vi "Filter Wheel GUI.vi"(9 "Standalone":bool=TRUE, 10 "Init Data":variant, 11 "Filter Wheel name":string="Default") -> ()   [LabVIEW 2021]
uses:
  Filter Wheel Arduino Control/Filter Wheel Arduino Command cluster.ctl
  typedefs/CC enum Operation Mode.ctl
  Filter Wheel Arduino Control/Filter Wheel Arduino Homing cluster.ctl
  Filter Wheel Object/Filter Wheel.lvclass
  Filter Wheel configuration.ctl
  Filter Wheel Object/Filter Wheel Details.ctl
  Subsystems/SS typedef cluster Instrument Command Queue Data.ctl
  Subsystems/SS cluster Data Queue type.ctl
  FW cmd Q Move Parameters.ctl
  <vilib>/Utility/miscctls.llb/LVRowAndColumnTypeDef.ctl
  FW cluster Status.ctl
  FW enum status.ctl
  Filter Wheel Object/Filter Wheel.lvclass/Filter Wheel.ctl
  hk-channel-class/HK Item/HK Channel Units and Setup.ctl
  hk-channel-class/HK Item/HK Channel enum Data Type.ctl
  hk-channel-class/HK Item/HK Item.lvclass
  hk-channel-class/HK Item/HK Channel cluster Telemetry Data.ctl
  FW cmd Q Move Position Parameters.ctl
  typedefs/CC cluster Alarm Data.ctl
  Filter Wheel Simulator/Filter Wheel Simulator.lvclass
  C:/Development/prime/Prime-RIMAS/Filter Wheel/Filter Wheel Object/Filter Wheel.lvclass
  Filter Wheel Simulator/Filter Wheel Simulator.lvclass/Filter Wheel Simulator.ctl
  Filter Wheel Arduino Control/FW Arduino Control.lvclass
panel:
  out "Messages":string
  in  "Mode":T1
  in  "Tab Control":T2(tab)
  out "Wheel Name":string
  out "Moving Message":string="Filter Wheel Moving...."
  in  "Error":bool
  out "Homed":bool[](array[boolean])
  in  "Wheel To Home":u16(ring) items=["InnerWheel", "OuterWheel"]
  in  "STOP":bool
  out "Connected":bool
  in  "Filter Wheel Displays":T3 {"Gauge 0" scale=0.0..3.0; "Gauge 4" scale=0.0..7.0; "Gauge 3" scale=0.0..5.0; "Gauge 2" scale=0.0..3.0; "Gauge 5" scale=0.0..32768.0; "Gauge 8" scale=0.0..32768.0; "Gauge 6" scale=0.0..32768.0; "Gauge 7" scale=0.0..32768.0}
  in  "Home":bool
  in  "Alarms?":bool=TRUE
  in  "Default Speed":u16=200 min=20 max=4000 step=10
  in  "Movement Parameters":T4
  in  "Sim Velocity (steps/sec)":i32
  in  "Connect":bool
  in  "Serial Port":refnum<visa-resource-name>="COM11"
  in  "Simulate":bool
  in  "Close":bool
  in  "Filter Wheel Table":cluster{i32[], "Dir":bool}[][](array[cluster])=[[{[], "Dir"=TRUE}, {[2800], "Dir"=TRUE}, {[2800, 2800], "Dir"=TRUE}, {[950, 1850], "Dir"=FALSE}], [{[2800], "Dir"=FALSE}, {[], "Dir"=TRUE}, {[2800], "Dir"=TRUE}, {[2800, 2800], "Dir"=TRUE}], [{[2800, 2800], "Dir"=FALSE}, {[2800], "Dir"=FALSE}, {[], "Dir"=TRUE}, {[2800], "Dir"=TRUE}], [{[2800, 2800], "Dir"=TRUE}, {[2800, 2800], "Dir"=FALSE}, {[2800], "Dir"=FALSE}, {[], "Dir"=TRUE}]]
  in  "Open Arduino Log":bool
  out "Moving":bool[](array[boolean])
  out "Last Move Positions":u32[](array[numeric])
  out "On the notch":bool[](array[boolean])
  in  "Filter Wheel Settings":T5={"Direction"=TRUE, "NUMBER OF  STEPS"=2900, "SPEED STEPS/SEC"=200, "ACC/DECEL STEPS/SEC^2"=4000, "Move mode"=0, "EN/DIS?"=TRUE, "delay before \nread (ms)"=750, "Timeout before \nstop (ms)"=13000} {"Move mode" items=["Relative steps ##", "Search switch"]; "ACC/DECEL STEPS/SEC^2" max=4000; "SPEED STEPS/SEC" min=20 max=4000 step=10}
  in  "MOTOR NUMBER":u8 max=3 step=1
  in  "Command Preview":string
  out "Response":string
  in  "Send Command":bool
  in  "Read":bool
  in  "Restore Defaults":bool
  in  "Remove Pos":bool
  in  "Add Pos":bool
  in  "Save Button":bool
  in  "Remove Fw":bool
  in  "Add Fw":bool
  in  "Wheels":i32(listbox)
  in  "Positions":i32(listbox)
  # "Click for info"
  # "Invalid combos defined here"
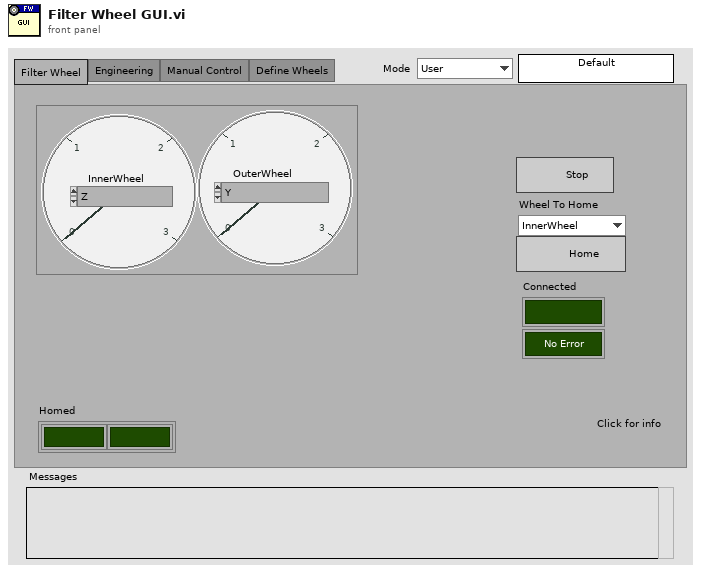
[diagram p1: front panel]
types:
  T1 = typedef "CC enum Operation Mode.ctl" = enum16{"User", "Engineering"}
  T2 = enum32{"Filter Wheel", "Engineering", "Manual Control", "Define Wheels"}
  T3 = cluster{"Gauge 0":i32, "Gauge 2":i32, "Gauge 3":i32, "Gauge 4":i32, "Gauge 5":i32, "Gauge 6":i32, "Gauge 7":i32, "Gauge 8":i32, "Position 0":i32, "Position 1":i32, "Position 2":i32, "Position 3":i32}
  T4 = typedef "Filter Wheel Arduino Homing cluster.ctl" = cluster{"Direction (F: CW)":bool, "Speed":i32, "Accel":i32, "Min Distance":i32, "Short Leg":i32, "Error Cnts":i32}
  T5 = typedef "Filter Wheel Arduino Command cluster.ctl" = cluster{"Direction":bool, "NUMBER OF  STEPS":u32, "SPEED STEPS/SEC":u16, "ACC/DECEL STEPS/SEC^2":u16, "Move mode":u16, "EN/DIS?":bool, "delay before \nread (ms)":u32, "Timeout before \nstop (ms)":u32}
  T6 = typedef "SS typedef cluster Instrument Command Queue Data.ctl" = cluster{"Cmd":string, "Parameters":variant}
  T7 = typedef "Filter Wheel.lvclass/Filter Wheel configuration.ctl" = cluster{"Num Wheels":i32, "Filters":T8[], "Invalid Combinations":i32[][], "Addr":refnum<visa-resource-name>, "Name":string, "Simulate":bool, "Homing Parameters":T4, "Default Speed":u16}
  T8 = typedef "Filter Wheel.lvclass/Filter Wheel Details.ctl" = cluster{"Names":string[], "Relative Position":i32[], "Wheel Name":string}
  T9 = typedef "FW cmd Q Move Parameters.ctl" = cluster{"Wheel ID":i32, "Position":i32}
  T10 = typedef "LVRowAndColumnTypeDef.ctl" = cluster{"Row":i32, "Column":i32}
  T11 = typedef "FW cluster Status.ctl" = cluster{"State":T12, "Positions":i32[], "Names":string[], "Notch":bool[], "Moving":bool[]}
  T12 = typedef "FW enum status.ctl" = enum16{"Initializing", "Moving", "Move Complete", "Error"}
  T13 = cluster{"state":refnum<user-event>, "Filter Wheel ref":refnum<class "Filter Wheel.lvclass">, "Filter Wheel Info":T7, "FW names":string[], "Pos Names":cluster{"Table":string[][]}[], "cmd q":refnum<queue>, "Cmd":T6, "Data Q":refnum<queue>, "Move":T9, "error":errorcluster, "next poll":timestamp, "FW refs":refnum<vi>[], "Wheel":i32, "Coords":T10, "Motor #":u8, "fw name":string, "Simulate":bool, "ch names":string[][], "FW Status":T11, "Error State":string, "Name":string, "Period":dbl}
  T14 = typedef "HK Item.lvclass/HK Channel Units and Setup.ctl" = cluster{"Unit Type":string, "Units":string, "Configuration":string, "Digits":i32, "Data Type":T15, "Exponential?":bool, "Source":string}
  T15 = typedef "HK Item.lvclass/HK Channel enum Data Type.ctl" = enum16{"Floating Point", "Integer", "Enum", "String", "Waveform", "File"}
  T16 = typedef "SS cluster Data Queue type.ctl" = cluster{"Source":string, "Type":string, "Data":variant}
  T17 = typedef "FW cmd Q Move Position Parameters.ctl" = cluster{"Position Names":string[]}
  T18 = enum32{"Page Enabled", "Page Disabled", "Page Disabled & Grayed"}
  T19 = typedef "CC cluster Alarm Data.ctl" = cluster{"Measured Value":dbl, "Alarm Low":dbl, "Alarm High":dbl, "Message":string, "Source":string}
  T20 = typedef "HK Item.lvclass/HK Channel cluster Telemetry Data.ctl" = cluster{"Ch Names":string[], "Ch Values":dbl[], "Timestamp":timestamp, "Data Type":T15}
  T21 = cluster{"Gauge 0":bool, "Gauge 2":bool, "Gauge 3":bool, "Gauge 4":bool, "Gauge 5":bool, "Gauge 6":bool, "Gauge 7":bool, "Gauge 8":bool, "Position 0":bool, "Position 1":bool, "Position 2":bool, "Position 3":bool}
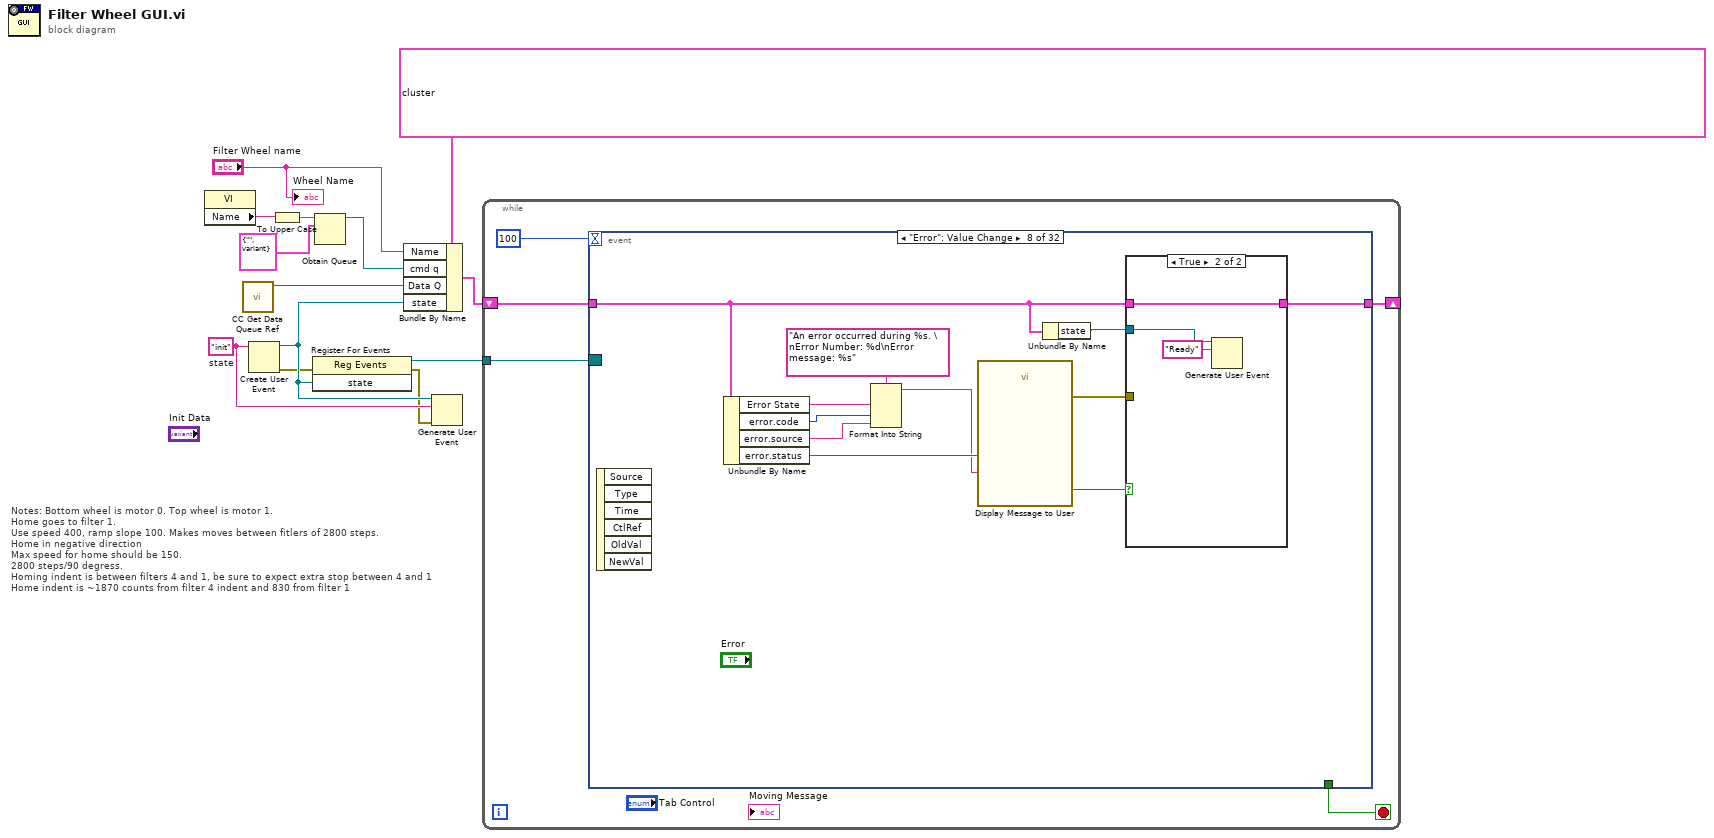
[diagram p0: block diagram]
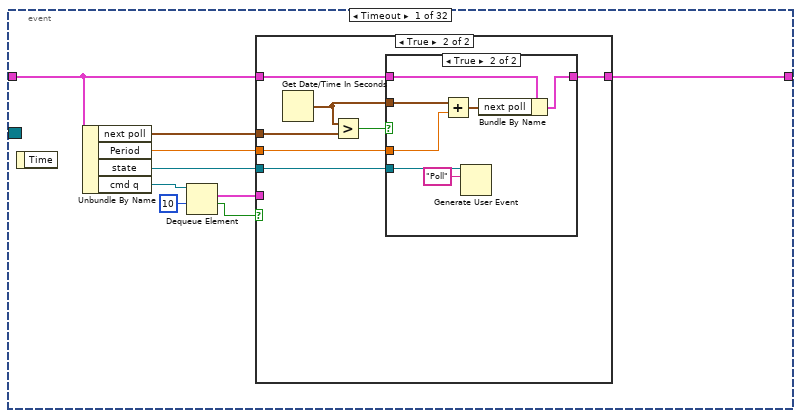
[diagram p2: hidden frame]
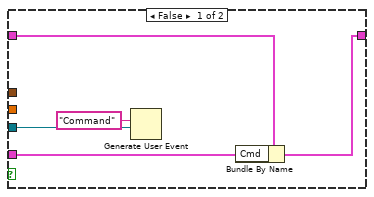
[diagram p3: hidden frame]
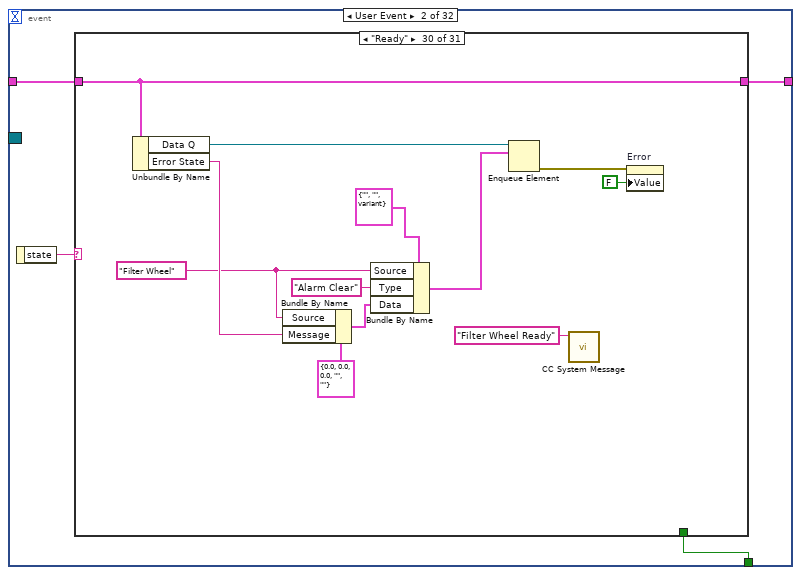
[diagram p5: hidden frame]
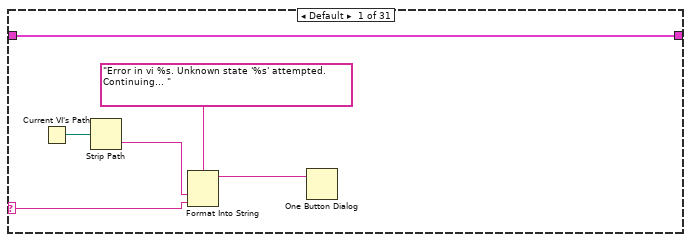
[diagram p6: hidden frame]
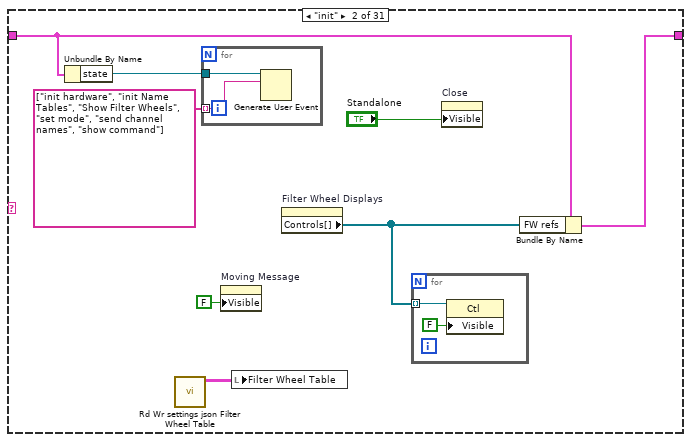
[diagram p7: hidden frame]
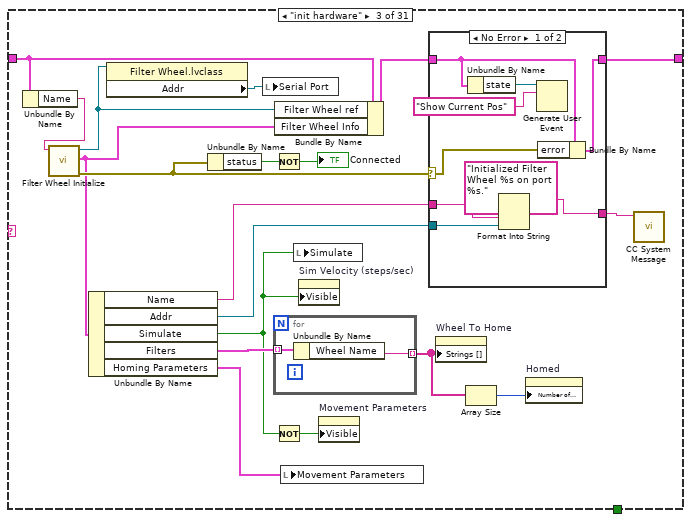
[diagram p8: hidden frame]
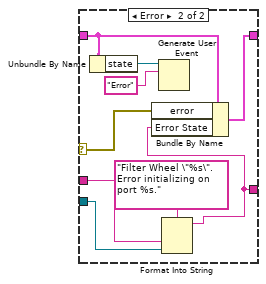
[diagram p9: hidden frame]
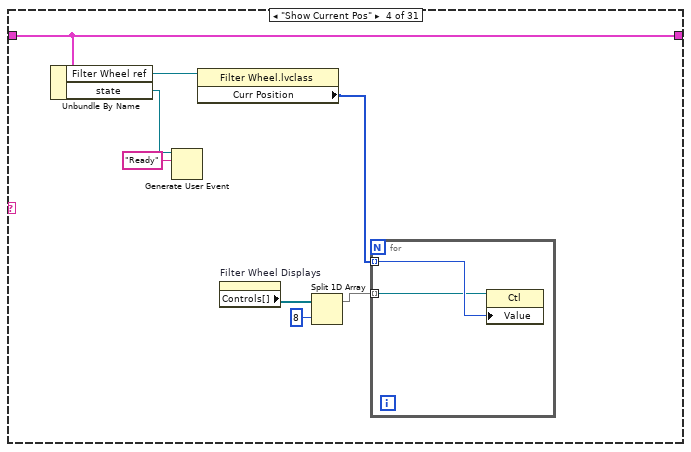
[diagram p10: hidden frame]
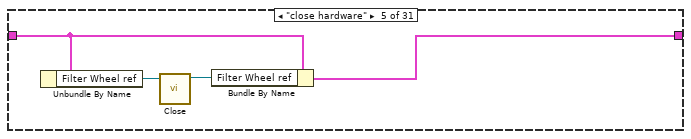
[diagram p11: hidden frame]
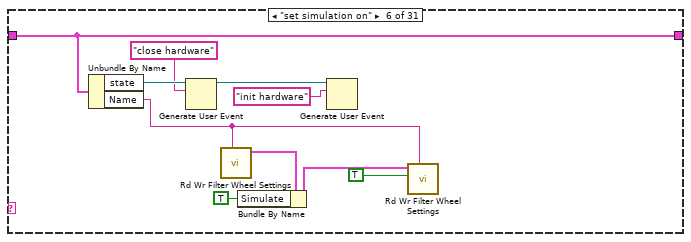
[diagram p12: hidden frame]
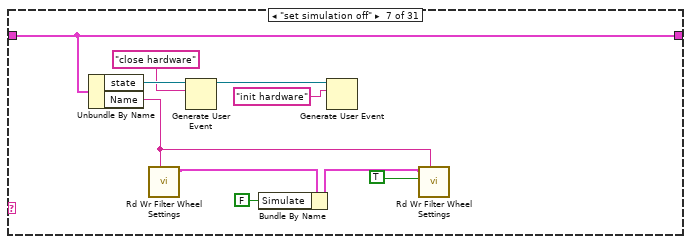
[diagram p13: hidden frame]
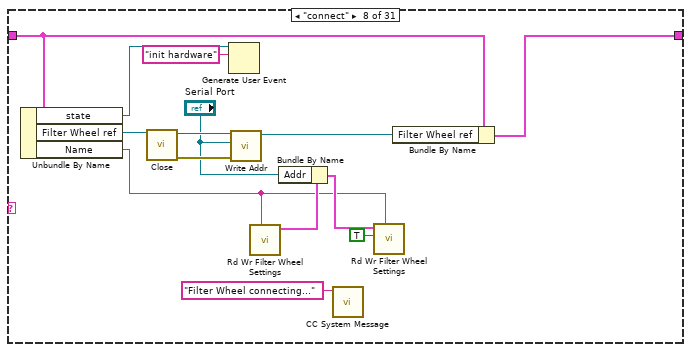
[diagram p14: hidden frame]
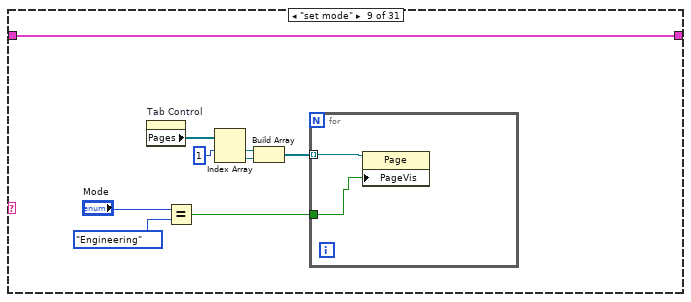
[diagram p15: hidden frame]
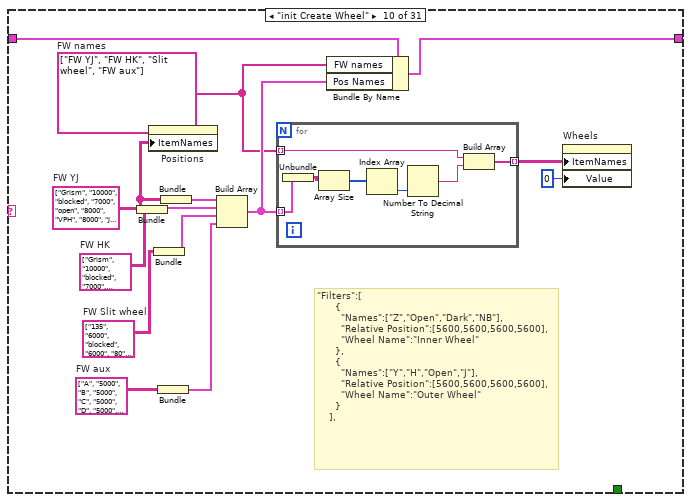
[diagram p16: hidden frame]
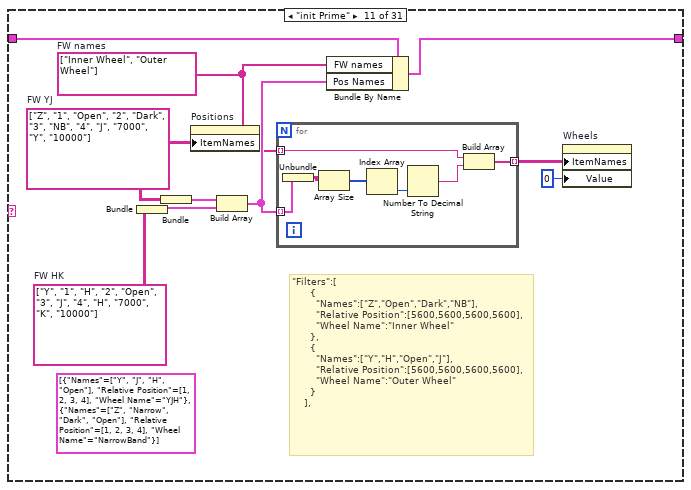
[diagram p17: hidden frame]
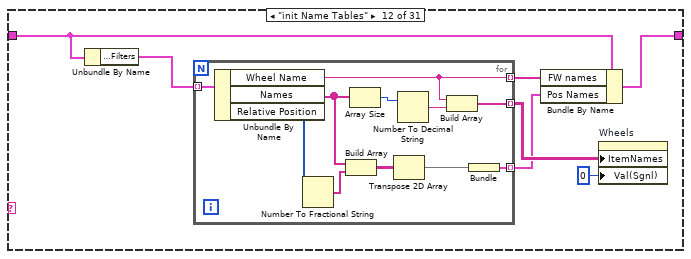
[diagram p18: hidden frame]
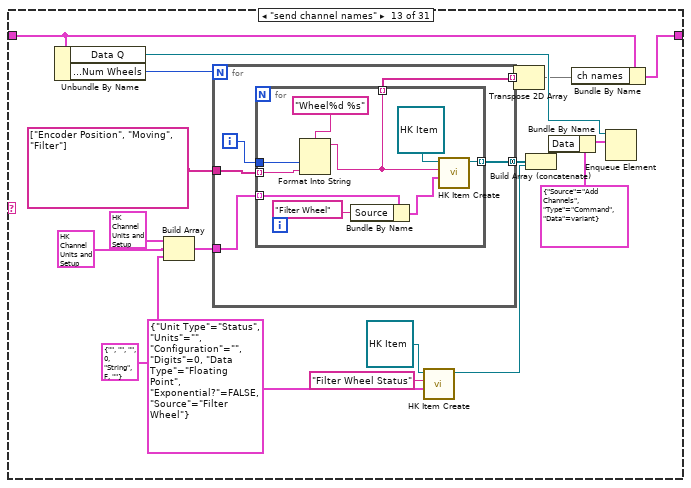
[diagram p19: hidden frame]
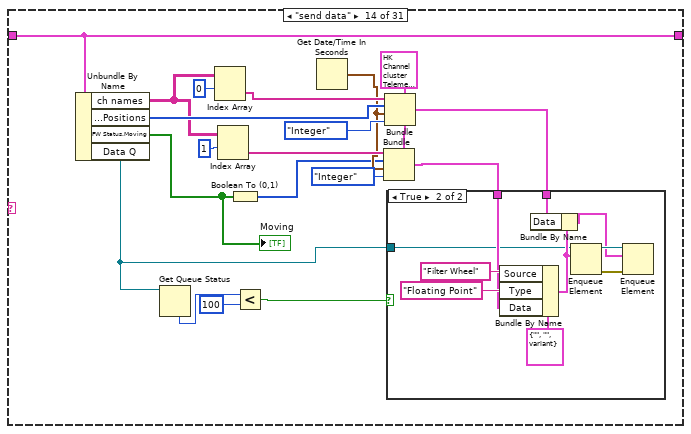
[diagram p20: hidden frame]
diagram:
  w9 = "init"  # state
  # "Notes: Bottom wheel is motor 0. Top wheel is motor 1.\nHome goes to filter 1. \nUse speed 400, ramp slope 100. Makes moves between fitlers of 2800 steps.\nHome in negative direction\nMax speed for home should be 150.\n2800 steps/90 degress.\nHoming indent is between filters 4 and 1, be sure to expect extra stop between 4 and 1\nHome indent is ~1870 counts from filter 4 indent and 830 from filter 1"
  n1 = property class="VI"() -> ("Name"=w5:string)  [unwired: 2 in, 2 out]
  n2 = call "CC Get Data Queue Ref.vi"() -> ("Data Q"=w6:refnum<queue>)  [unwired: 10 in, 1 out]
  n3 = Create User Event(user event datatype=w9) -> (user event=w11:refnum<user-event>, error out=w7:errorcluster)  [unwired: 1 in]
  n4 = To Upper Case(1:w5) -> (0:w4:string)
  n5 = register-events(error in=w7, w11) -> (reference out=w10:refnum<event-registration>, error out=w8:errorcluster)  [unwired: 1 in]
  n6 = Obtain Queue(name (unnamed)=w4, element data type=T6 {"Cmd"="", "Parameters"=variant}) -> (queue out=w2:refnum<queue>)  [unwired: 3 in, 2 out]
  n7 = Bundle By Name(cluster=T13 {"state"=refnum, "Filter Wheel ref"=refnum, "Filter Wheel Info"={"Num Wheels"=0, "Filters"=[], "Invalid Combinations"=[], "Addr"="", "Name"="", "Simulate"=FALSE, "Homing Parameters"={"Direction (F: CW)"=TRUE, "Speed"=150, "Accel"=400, "Min Distance"=2700, "Short Leg"=0, "Error Cnts"=0}, "Default Speed"=1000}, "FW names"=["FW YJ", "FW HK", "Slit wheel", "FW aux"], "Pos Names"=[], "cmd q"=refnum, "Cmd"={"Cmd"="", "Parameters"=variant}, "Data Q"=refnum, "Move"={"Wheel ID"=0, "Position"=0}, "error"={"status"=FALSE, "code"=0, "source"=""}, "next poll"=timestamp(0 s since 1904-01-01), "FW refs"=[], "Wheel"=0, "Coords"={"Row"=0, "Column"=0}, "Motor #"=0, "fw name"="", "Simulate"=TRUE, "ch names"=[], "FW Status"={"State"=enum."Move Complete", "Positions"=[], "Names"=[], "Notch"=[], "Moving"=[FALSE, FALSE]}, "Error State"="", "Name"="PRIME", "Period"=1.0}, "Name"="Filter Wheel name", "cmd q"=w2, "Data Q"=w6, "state"=w11) -> (w12:T13)
  n8 = Generate User Event(user event=w11, event data cluster=w9, error in=w8) -> ()  [unwired: 1 in, 2 out]
  n9 = while {
    tunnel: w10 -> [w18]
    shift-right: [w17] -> _
    shift-left: w12 -> [w14]
    stop <- w16 stop-if-true
    n10 = event shown="[7] \"Error\": Value Change" {
      selector: w18 -> [_ _ _ _ _ _ _ _ _ _ _ _ _ _ _ _ _ _ _ _ _ _ _ _ _ _ _ _ _ _ _ _]
      dyn-events: _ -> [_ _ _ _ _ _ _ _ _ _ _ _ _ _ _ _ _ _ _ _ _ _ _ _ _ _ _ _ _ _ _ _]
      timeout: 100 -> [_ _ _ _ _ _ _ _ _ _ _ _ _ _ _ _ _ _ _ _ _ _ _ _ _ _ _ _ _ _ _ _]
      tunnel: w14 -> [w22 w50 w572 w574 w583 w586 w589 w591 w613 w620 w629 w635 w636 w651 w654 w657 w658 w663 w666 w675 w679 w685 w692 w697 w713 w735 w744 w750 w773 w784 w804 w808]
      tunnel: [w21 w49 w572 w573 w583 w586 w589 w594 w614 w621 w629 w635 w637 w651 w654 w657 w659 w663 w666 w676 w680 w686 w693 w698 w714 w736 w745 w751 w774 w785 w804 w808] -> w17
      tunnel: [_ w48 _ _ _ _ _ _ _ _ _ _ _ _ _ _ _ _ _ _ _ _ _ _ _ _ _ _ _ _ _ _] -> w16
      event Timeout {
        n11 = event-data() -> ()  [unwired: 1 in, 1 out]
        n12 = Unbundle By Name(w22) -> ("next poll"=w20:timestamp, "Period"=w19:dbl, "state"=w23:refnum<user-event>, "cmd q"=w27:refnum<queue>)
        n13 = Dequeue Element(queue=w27, timeout in ms (-1)=10) -> (element=w24:T6, timed out?=w25:bool)  [unwired: 1 in, 2 out]
        n14 = case shown="True" w25 {
          tunnel: w24 -> [w29 _]
          tunnel: w23 -> [w32 w36]
          tunnel: w22 -> [w30 w37]
          tunnel: [w28 w34] -> w21
          tunnel: w20 -> [_ w39]
          tunnel: w19 -> [_ w33]
          frame False {
            n15 = Generate User Event(user event=w32, event data cluster="Command" ("event data")) -> ()  [unwired: 2 in, 2 out]
            n16 = Bundle By Name(cluster=w30, "Cmd"=w29) -> (w28:T13)
          }
          frame True {
            n17 = Get Date/Time In Seconds() -> (seconds since 1Jan1904=w35:timestamp)
            n18 = Greater?(x=w35, y=w39) -> (0:w38:bool)
            n19 = case shown="True" w38 {
              tunnel: w37 -> [w40 w47]
              tunnel: w36 -> [_ w46]
              tunnel: w35 -> [_ w45]
              tunnel: [w40 w43] -> w34
              tunnel: w33 -> [_ w41]
              frame False {
              }
              frame True {
                n20 = Add(x=w45, y=w41) -> (x+y=w44:timestamp)
                n21 = Generate User Event(user event=w46, event data cluster="Poll" ("event data")) -> ()  [unwired: 2 in, 2 out]
                n22 = Bundle By Name(cluster=w47, "next poll"=w44) -> (w43:T13)
              }
            }
          }
        }
      }
      event User Event {
        n23 = event-data() -> ("state"=w51:string)  [unwired: 1 in]
        n24 = case shown="\"Ready\"" w51 {
          selector: w51 -> [w56 _ _ _ _ _ _ _ _ _ _ _ _ _ _ _ _ _ _ _ _ _ _ _ _ _ _ _ _ _ _]
          tunnel: w50 -> [w52 w64 w75 w116 w119 w131 w141 w152 w165 w168 w189 w210 w231 w275 w290 w300 w313 w322 w364 w422 w445 w473 w489 w502 w518 w526 w533 w540 w545 w566 w569]
          tunnel: [w52 w65 w87 w116 w120 w131 w141 w153 w165 w169 w190 w211 w232 w275 w290 w300 w313 w323 w373 w423 w463 w472 w490 w503 w519 w527 w533 w540 w546 w566 w569] -> w49
          tunnel: [_ _ _ _ _ _ _ _ _ _ _ _ _ _ _ _ _ _ _ _ _ _ _ _ _ _ _ _ _ _ TRUE] -> w48
          frame Default {
            n25 = Current VI's Path() -> (path=w55:path)
            n26 = Strip Path(path=w55) -> (name=w54:string)  [unwired: 1 out]
            n27 = Format Into String(format string="Error in vi %s. Unknown state '%s' attempted. Continuing... ", w54, w56) -> (resulting string=w53:string)  [unwired: 2 in, 1 out]
            n28 = One Button Dialog(message=w53) -> ()  [unwired: 1 in, 1 out]
          }
          frame "init" {
            n29 = Unbundle By Name(w64) -> ("state"=w63:refnum<user-event>)
            n30 = call "Rd Wr settings json Filter Wheel Table.vi"() -> ("Filter Wheel Table"=w58:cluster{i32[], bool}[][])  [unwired: 10 in, 1 out]
            n31 = for {
              tunnel: w63 -> [w69]
              tunnel: string[] ["init hardware", "init Name Tables", "Show Filter Wheels", "set mode", "send channel names", "show command"] -> [w68] mode=indexing
              n32 = Generate User Event(user event=w69, event data cluster=w68) -> ()  [unwired: 2 in, 2 out]
            }
            n33 = property on="Moving Message" class="Str"("Visible"=FALSE) -> ()  [unwired: 2 in, 2 out]
            n34 = local write "Filter Wheel Table"(w58) -> ()
            n35 = property on="Filter Wheel Displays" class="Clust (strict)"() -> ("Controls[]"=w60:refnum<vi>[])  [unwired: 2 in, 2 out]
            n36 = for {
              tunnel: w60 -> [w67] mode=indexing
              n37 = property class="Ctl"(reference=w67, "Visible"=FALSE) -> ()  [unwired: 1 in, 2 out]
            }
            n38 = property on="Close" class="Bool"("Visible"="Standalone") -> ()  [unwired: 2 in, 2 out]
            n39 = Bundle By Name(cluster=w64, "FW refs"=w60) -> (w65:T13)
          }
          frame "init hardware" {
            n40 = Unbundle By Name(w75) -> ("Name"=w74:string)
            n41 = call "Filter Wheel Initialize.vi"("Wheel Name"=w74) -> ("error out"=w86:errorcluster, "Filter Wheel Info"=w83:T7, "Filter Wheel.lvclass"=w71:refnum<class "Filter Wheel.lvclass">)  [unwired: 8 in]
            n42 = Unbundle By Name(w83) -> ("Name"=w82:string, "Addr"=w81:refnum<visa-resource-name>, "Simulate"=w72:bool, "Filters"=w79:T8[], "Homing Parameters"=w78:T4)
            n43 = property class="Filter Wheel.lvclass"(reference=w71) -> ("Addr"=w70:refnum<visa-resource-name>)  [unwired: 1 in, 2 out]
            n44 = Unbundle By Name(w86) -> ("status"=w85:bool)
            n45 = local write "Serial Port"(w70) -> ()
            n46 = Not(x=w85) -> (.not. x?=→"Connected":bool)
            n47 = for {
              tunnel: [w89] -> w77 mode=indexing
              tunnel: w79 -> [w90] mode=indexing
              n48 = Unbundle By Name(w90) -> ("Wheel Name"=w89:string)
            }
            n49 = Not(x=w72) -> (.not. x?=w73:bool)
            n50 = Bundle By Name(cluster=w75, "Filter Wheel ref"=w71, "Filter Wheel Info"=w83) -> (w88:T13)
            n51 = local write "Movement Parameters"(w78) -> ()
            n52 = local write "Simulate"(w72) -> ()
            n53 = property on="Sim Velocity (steps/sec)" class="DigNum (strict)"("Visible"=w72) -> ()  [unwired: 2 in, 2 out]
            n54 = property on="Movement Parameters" class="Clust (strict)"("Visible"=w73) -> ()  [unwired: 2 in, 2 out]
            n55 = case shown="No Error" w86 {
              selector: w86 -> [w93 w107]
              tunnel: [w92 w106] -> w87
              tunnel: w88 -> [w91 w105]
              tunnel: w82 -> [w98 w102]
              tunnel: w81 -> [w97 w101]
              tunnel: [w96 w100] -> w80
              frame No Error {
                n56 = Unbundle By Name(w91) -> ("state"=w94:refnum<user-event>)
                n57 = Format Into String(format string="Initialized Filter Wheel %s on port %s.", w98, w97) -> (resulting string=w96:string)  [unwired: 2 in, 1 out]
                n58 = Generate User Event(user event=w94, event data cluster="Show Current Pos" ("event data")) -> ()  [unwired: 2 in, 2 out]
                n59 = Bundle By Name(cluster=w91, "error"=w93) -> (w92:T13)
              }
              frame Error {
                n60 = Unbundle By Name(w105) -> ("state"=w104:refnum<user-event>)
                n61 = Generate User Event(user event=w104, event data cluster="Error" ("event data")) -> ()  [unwired: 2 in, 2 out]
                n62 = Format Into String(format string="Filter Wheel \"%s\". Error initializing on port %s.", w102, w101) -> (resulting string=w100:string)  [unwired: 2 in, 1 out]
                n63 = Bundle By Name(cluster=w105, "error"=w107, "Error State"=w100) -> (w106:T13)
              }
            }
            n64 = property on="Wheel To Home" class="Ring (strict)"("Strings []"=w77) -> ()  [unwired: 2 in, 2 out]
            n65 = Array Size(array=w77) -> (size(s)=w76:i32)
            n66 = property on="Homed" class="Arr (strict)"("Number of Columns"=w76) -> ()  [unwired: 2 in, 2 out]
            n67 = call "CC System Message.vi"("Message"=w80) -> ()  [unwired: 10 in, 1 out]
          }
          frame "Show Current Pos" {
            n68 = Unbundle By Name(w116) -> ("Filter Wheel ref"=w115:refnum<class "Filter Wheel.lvclass">, "state"=w114:refnum<user-event>)
            n69 = Generate User Event(user event=w114, event data cluster="Ready" ("event data")) -> ()  [unwired: 2 in, 2 out]
            n70 = property class="Filter Wheel.lvclass"(reference=w115) -> ("Curr Position"=w110:i32[])  [unwired: 1 in, 2 out]
            n71 = property on="Filter Wheel Displays" class="Clust (strict)"() -> ("Controls[]"=w112:refnum<vi>[])  [unwired: 2 in, 2 out]
            n72 = Split 1D Array(array=w112, index=8) -> (first subarray=w109:refnum<vi>[])  [unwired: 1 out]
            n73 = for {
              tunnel: w110 -> [w118] mode=indexing
              tunnel: w109 -> [w117] mode=indexing
              n74 = property class="Ctl"(reference=w117, "Value"=w118) -> ()  [unwired: 1 in, 2 out]
            }
          }
          frame "close hardware" {
            n75 = Unbundle By Name(w119) -> ("Filter Wheel ref"=w122:refnum<class "Filter Wheel.lvclass">)
            n76 = call-dynamic "Close.vi"("Filter Wheel in"=w122) -> ("Filter Wheel out"=w121:refnum<class "Filter Wheel.lvclass">)  [unwired: 9 in, 1 out]
            n77 = Bundle By Name(cluster=w119, "Filter Wheel ref"=w121) -> (w120:T13)
          }
          frame "set simulation on" {
            n78 = Unbundle By Name(w131) -> ("state"=w130:refnum<user-event>, "Name"=w123:string)
            n79 = Generate User Event(user event=w130, event data cluster="close hardware" ("event data")) -> (user event out=w129:refnum<user-event>)  [unwired: 2 in, 1 out]
            n80 = call "Rd Wr Filter Wheel Settings.vi"("Wheel Name"=w123) -> ("Filter Wheel Settings"=w126:T7)  [unwired: 9 in, 1 out]
            n81 = Bundle By Name(cluster=w126, "Simulate"=TRUE) -> (w125:T7)
            n82 = Generate User Event(user event=w129, event data cluster="init hardware" ("event data")) -> ()  [unwired: 2 in, 2 out]
            n83 = call "Rd Wr Filter Wheel Settings.vi"("Wheel Name"=w123, "Write? (F:Read)"=TRUE, "Filter Wheel Settings"=w125) -> ()  [unwired: 7 in, 2 out]
          }
          frame "set simulation off" {
            n84 = Unbundle By Name(w141) -> ("state"=w140:refnum<user-event>, "Name"=w133:string)
            n85 = call "Rd Wr Filter Wheel Settings.vi"("Wheel Name"=w133) -> ("Filter Wheel Settings"=w136:T7)  [unwired: 9 in, 1 out]
            n86 = Generate User Event(user event=w140, event data cluster="close hardware" ("event data")) -> (user event out=w139:refnum<user-event>)  [unwired: 2 in, 1 out]
            n87 = Bundle By Name(cluster=w136, "Simulate"=FALSE) -> (w135:T7)
            n88 = Generate User Event(user event=w139, event data cluster="init hardware" ("event data")) -> ()  [unwired: 2 in, 2 out]
            n89 = call "Rd Wr Filter Wheel Settings.vi"("Wheel Name"=w133, "Write? (F:Read)"=TRUE, "Filter Wheel Settings"=w135) -> ()  [unwired: 7 in, 2 out]
          }
          frame "connect" {
            n90 = Unbundle By Name(w152) -> ("state"=w150:refnum<user-event>, "Filter Wheel ref"=w156:refnum<class "Filter Wheel.lvclass">, "Name"=w143:string)
            n91 = call-dynamic "Close.vi"("Filter Wheel in"=w156) -> ("error out"=w154:errorcluster, "Filter Wheel out"=w155:refnum<class "Filter Wheel.lvclass">)  [unwired: 9 in]
            n92 = Generate User Event(user event=w150, event data cluster="init hardware" ("event data")) -> ()  [unwired: 2 in, 2 out]
            n93 = call "Write Addr.vi"("error in (no error)"=w154, "Addr"="Serial Port", "Filter Wheel in"=w155) -> ("Filter Wheel out"=w151:refnum<class "Filter Wheel.lvclass">)  [unwired: 7 in, 1 out]
            n94 = call "Rd Wr Filter Wheel Settings.vi"("Wheel Name"=w143) -> ("Filter Wheel Settings"=w148:T7)  [unwired: 9 in, 1 out]
            n95 = Bundle By Name(cluster=w148, "Addr"="Serial Port") -> (w146:T7)
            n96 = call "CC System Message.vi"("Message"="Filter Wheel connecting...") -> ()  [unwired: 10 in, 1 out]
            n97 = call "Rd Wr Filter Wheel Settings.vi"("Wheel Name"=w143, "Write? (F:Read)"=TRUE, "Filter Wheel Settings"=w146) -> ()  [unwired: 7 in, 2 out]
            n98 = Bundle By Name(cluster=w152, "Filter Wheel ref"=w151) -> (w153:T13)
          }
          frame "set mode" {
            n99 = property on="Tab Control" class="TabCtl (strict)"() -> ("Pages"=w164:refnum<vi>[])  [unwired: 2 in, 2 out]
            n100 = Equal?(x="Mode", y=CC_enum_Operation_Mode."Engineering") -> (x = y?=w157:bool)
            n101 = Index Array(array=w164, index #1=1 ("index")) -> (element #1=w162:refnum<vi>, element #2=w161:refnum<vi>)  [unwired: 1 in]
            n102 = Build Array(w162, w161) -> (w160:refnum<vi>[])
            n103 = for {
              tunnel: w160 -> [w167] mode=indexing
              tunnel: w157 -> [w166]
              n104 = property class="Page"(reference=w167, "PageVis"=w166) -> ()  [unwired: 1 in, 2 out]
            }
          }
          frame "init Create Wheel" {
            w170 = string[] ["FW YJ", "FW HK", "Slit wheel", "FW aux"]  # FW names
            w178 = string[][] [["Grism", "10000"], ["blocked", "7000"], ["open", "8000"], ["VPH", "8000"], ["J", "7000"], ["Y", "10000"]]  # FW YJ
            w181 = string[][] [["Grism", "10000"], ["blocked", "7000"], ["open", "8000"], ["VPH", "8000"], ["H", "7000"], ["K", "10000"]]  # FW HK
            w173 = string[][] [["135", "6000"], ["blocked", "6000"], ["80", "7000"], ["open 1", "7000"], ["250", "7000"], ["open", "7000"]]  # FW Slit wheel
            w180 = string[][] [["A", "5000"], ["B", "5000"], ["C", "5000"], ["D", "5000"], ["E", "5000"], ["F", "5000"], ["G", "5000"], ["H", "5000"]]  # FW aux
            # "\"Filters\":[\n      {\n        \"Names\":[\"Z\",\"Open\",\"Dark\",\"NB\"],\n        \"Relative Position\":[5600,5600,5600,5600],\n        \"Wheel Name\":\"Inner Wheel\"\n      },\n      {\n        \"Names\":[\"Y\",\"H\",\"Open\",\"J\"],\n        \"Relative Position\":[5600,5600,5600,5600],\n        \"Wheel Name\":\"Outer Wheel\"\n      }\n    ],"
            n105 = Bundle("FW HK"=w181) -> (w175:cluster{"FW HK":string[][]})  [unwired: 1 in]
            n106 = property on="Positions" class="MCListbox (strict)"("ItemNames"=w178) -> ()  [unwired: 2 in, 2 out]
            n107 = Bundle("FW Slit wheel"=w173) -> (w174:cluster{"FW Slit wheel":string[][]})  [unwired: 1 in]
            n108 = Bundle("FW aux"=w180) -> (w172:cluster{"FW aux":string[][]})  [unwired: 1 in]
            n109 = Bundle("FW YJ"=w178) -> (w176:cluster{"FW YJ":string[][]})  [unwired: 1 in]
            n110 = Build Array(w176, w175, w174, w172) -> (w171:cluster{"FW aux":string[][]}[])
            n111 = for {
              tunnel: w171 -> [w188] mode=indexing
              tunnel: w170 -> [w184] mode=indexing
              tunnel: [w183] -> w179 mode=indexing
              n112 = Unbundle(w188) -> ("FW aux"=w182:string[][])
              n113 = Array Size(array=w182) -> (size(s)=w187:i32[])
              n114 = Index Array(array=w187) -> (element=w186:i32)  [unwired: 1 in]
              n115 = Number To Decimal String(number=w186) -> (decimal integer string=w185:string)  [unwired: 1 in]
              n116 = Build Array(w184, w185) -> (w183:string[])
            }
            n117 = Bundle By Name(cluster=w168, "FW names"=w170, "Pos Names"=w171) -> (w169:T13)
            n118 = property on="Wheels" class="MCListbox (strict)"("ItemNames"=w179, "Value"=0 ("Wheels")) -> ()  [unwired: 2 in, 2 out]
          }
          frame "init Prime" {
            (unwired) T8[] [{"Names"=["Y", "J", "H", "Open"], "Relative Position"=[1, 2, 3, 4], "Wheel Name"="YJH"}, {"Names"=["Z", "Narrow", "Dark", "Open"], "Relative Position"=[1, 2, 3, 4], "Wheel Name"="NarrowBand"}] ("Filter Wheel Info.Filters")
            w191 = string[] ["Inner Wheel", "Outer Wheel"]  # FW names
            w196 = string[][] [["Z", "1"], ["Open", "2"], ["Dark", "3"], ["NB", "4"], ["J", "7000"], ["Y", "10000"]]  # FW YJ
            w198 = string[][] [["Y", "1"], ["H", "2"], ["Open", "3"], ["J", "4"], ["H", "7000"], ["K", "10000"]]  # FW HK
            # "\"Filters\":[\n      {\n        \"Names\":[\"Z\",\"Open\",\"Dark\",\"NB\"],\n        \"Relative Position\":[5600,5600,5600,5600],\n        \"Wheel Name\":\"Inner Wheel\"\n      },\n      {\n        \"Names\":[\"Y\",\"H\",\"Open\",\"J\"],\n        \"Relative Position\":[5600,5600,5600,5600],\n        \"Wheel Name\":\"Outer Wheel\"\n      }\n    ],"
            n119 = Bundle("FW HK"=w198) -> (w193:cluster{"FW HK":string[][]})  [unwired: 1 in]
            n120 = Bundle("FW YJ"=w196) -> (w194:cluster{"FW YJ":string[][]})  [unwired: 1 in]
            n121 = property on="Positions" class="MCListbox (strict)"("ItemNames"=w196) -> ()  [unwired: 2 in, 2 out]
            n122 = Build Array(w194, w193) -> (w192:cluster{"FW HK":string[][]}[])
            n123 = for {
              tunnel: w192 -> [w205] mode=indexing
              tunnel: w191 -> [w201] mode=indexing
              tunnel: [w200] -> w197 mode=indexing
              n124 = Unbundle(w205) -> ("FW HK"=w199:string[][])
              n125 = Array Size(array=w199) -> (size(s)=w204:i32[])
              n126 = Index Array(array=w204) -> (element=w203:i32)  [unwired: 1 in]
              n127 = Number To Decimal String(number=w203) -> (decimal integer string=w202:string)  [unwired: 1 in]
              n128 = Build Array(w201, w202) -> (w200:string[])
            }
            n129 = Bundle By Name(cluster=w189, "FW names"=w191, "Pos Names"=w192) -> (w190:T13)
            n130 = property on="Wheels" class="MCListbox (strict)"("ItemNames"=w197, "Value"=0 ("Wheels")) -> ()  [unwired: 2 in, 2 out]
          }
          frame "init Name Tables" {
            n131 = Unbundle By Name(w210) -> ("Filter Wheel Info.Filters"=w209:T8[])
            n132 = for {
              tunnel: w209 -> [w223] mode=indexing
              tunnel: [w220] -> w208 mode=indexing
              tunnel: [w219] -> w207 mode=indexing
              tunnel: [w214] -> w206 mode=indexing
              n133 = Unbundle By Name(w223) -> ("Wheel Name"=w220:string, "Names"=w216:string[], "Relative Position"=w218:i32[])
              n134 = Number To Fractional String(number=w218) -> (F-format string=w217:string[])  [unwired: 3 in]
              n135 = Build Array(w216, w217) -> (w215:string[][])
              n136 = Array Size(array=w216) -> (size(s)=w222:i32)
              n137 = Transpose 2D Array(2D array=w215) -> (transposed array=w213:string[][])
              n138 = Number To Decimal String(number=w222) -> (decimal integer string=w221:string)  [unwired: 1 in]
              n139 = Build Array(w220, w221) -> (w219:string[])
              n140 = Bundle(w213) -> (w214:cluster{string[][]})  [unwired: 1 in]
            }
            n141 = Bundle By Name(cluster=w210, "FW names"=w208, "Pos Names"=w206) -> (w211:T13)
            n142 = property on="Wheels" class="MCListbox (strict)"("ItemNames"=w207, "Val(Sgnl)"=0 ("Wheels")) -> ()  [unwired: 2 in, 2 out]
          }
          frame "send channel names" {
            n143 = Unbundle By Name(w231) -> ("Data Q"=w235:refnum<queue>, "Filter Wheel Info.Num Wheels"=w234:i32)
            n144 = Build Array(T14 {"Unit Type"="", "Units"="Counts", "Configuration"="", "Digits"=0, "Data Type"=enum."Integer", "Exponential?"=FALSE, "Source"=""} ("Channel Setup"), T14 {"Unit Type"="", "Units"="OnOff", "Configuration"="", "Digits"=0, "Data Type"=enum."Integer", "Exponential?"=FALSE, "Source"=""} ("Channel Setup"), T14 {"Unit Type"="", "Units"="", "Configuration"="", "Digits"=0, "Data Type"=enum."String", "Exponential?"=FALSE, "Source"=""} ("Channel Setup")) -> (w238:T14[])
            n145 = for {
              N: w234 -> [_]
              tunnel: string[] ["Encoder Position", "Moving", "Filter"] -> [w247]
              tunnel: w238 -> [w246]
              tunnel: [w245] -> w233 mode=concatenating
              tunnel: [w243] -> w230 mode=indexing
              i -> [w244]
              n146 = for {
                tunnel: w247 -> [w254] mode=indexing
                tunnel: w246 -> [w249] mode=indexing
                tunnel: [w253] -> w245 mode=indexing
                tunnel: w244 -> [w252]
                tunnel: [w251] -> w243 mode=indexing
                n147 = Format Into String(format string="Wheel%d %s", w252, w254) -> (resulting string=w251:string)  [unwired: 2 in, 1 out]
                n148 = Bundle By Name(cluster=w249, "Source"="Filter Wheel") -> (w250:T14)
                n149 = call-dynamic "HK Item Create.vi"("Channel Setup"=w250, "Name"=w251, "HK Item in"=refnum<class "HK Item.lvclass"> refnum) -> ("HK Item out"=w253:refnum<class "HK Item.lvclass">)  [unwired: 7 in, 1 out]
              }
            }
            n150 = call-dynamic "HK Item Create.vi"("Channel Setup"=T14 {"Unit Type"="Status", "Units"="", "Configuration"="", "Digits"=0, "Data Type"=enum."Floating Point", "Exponential?"=FALSE, "Source"="Filter Wheel"}, "Name"="Filter Wheel Status", "HK Item in"=refnum<class "HK Item.lvclass"> refnum) -> ("HK Item out"=w224:refnum<class "HK Item.lvclass">)  [unwired: 7 in, 1 out]
            n151 = Transpose 2D Array(2D array=w230) -> (transposed array=w229:string[][])
            n152 = Build Array (concatenate)(w233, w224) -> (w225:refnum<class "HK Item.lvclass">[])
            n153 = Bundle By Name(cluster=T16 {"Source"="Add Channels", "Type"="Command", "Data"=variant} ("element"), "Data"=w225) -> (w237:T16)
            n154 = Bundle By Name(cluster=w231, "ch names"=w229) -> (w232:T13)
            n155 = Enqueue Element(queue=w235, element=w237) -> ()  [unwired: 2 in, 3 out]
          }
          frame "send data" {
            w268 = T20 {"Ch Names"=[], "Ch Values"=[], "Timestamp"=timestamp(0 s since 1904-01-01), "Data Type"=enum."Floating Point"} ("cluster")
            n156 = Unbundle By Name(w275) -> ("ch names"=w269:string[][], "FW Status.Positions"=w271:i32[], "FW Status.Moving"=w257:bool[], "Data Q"=w262:refnum<queue>)
            "Moving" <- w257
            n157 = Get Queue Status(queue=w262) -> (# elements in queue=w261:i32)  [unwired: 2 in, 7 out]
            n158 = Index Array(array=w269, index (row)=0) -> (element=w272:string[])  [unwired: 1 in]
            n159 = Index Array(array=w269, index (row)=1) -> (element=w267:string[])  [unwired: 1 in]
            n160 = Boolean To (0,1)(Boolean=w257) -> (0, 1=w258:i16[])
            n161 = Less?(x=w261, y=100) -> (x < y?=w259:bool)
            n162 = Get Date/Time In Seconds() -> (seconds since 1Jan1904=w266:timestamp)
            n163 = Bundle(cluster=w268, "Ch Names"=w267, "Ch Values"=w258, "Timestamp"=w266, "Data Type"=HK_Channel_enum_Data_Type."Integer") -> (w264:T20)
            n164 = Bundle(cluster=w268, "Ch Names"=w272, "Ch Values"=w271, "Timestamp"=w266, "Data Type"=HK_Channel_enum_Data_Type."Integer") -> (w263:T20)
            n165 = case shown="True" w259 {
              tunnel: w264 -> [_ w282]
              tunnel: w263 -> [_ w279]
              tunnel: w262 -> [_ w276]
              frame False {
              }
              frame True {
                n166 = Bundle By Name(cluster=T16 {"Source"="", "Type"="", "Data"=variant} ("element"), "Source"="Filter Wheel", "Type"="Floating Point" ("Data Type"), "Data"=w282) -> (w280:T16)
                n167 = Bundle By Name(cluster=w280, "Data"=w279) -> (w278:T16)
                n168 = Enqueue Element(queue=w276, element=w280) -> (queue out=w281:refnum<queue>, error out=w277:errorcluster)  [unwired: 2 in, 1 out]
                n169 = Enqueue Element(queue=w281, element=w278, error in (no error)=w277) -> ()  [unwired: 1 in, 3 out]
              }
            }
          }
          frame "Show Tables" {
            n170 = Unbundle By Name(w290) -> ("FW names"=w289:string[], "Pos Names"=w288:cluster{"Table":string[][]}[])
            n171 = for {
              tunnel: w289 -> [w292] mode=indexing
              tunnel: w288 -> [w296] mode=indexing
              tunnel: [w291] -> w286 mode=indexing
              n172 = Unbundle By Name(w296) -> ("Table"=w295:string[][])
              n173 = Array Size(array=w295) -> (size(s)=w294:i32[])
              n174 = Number To Decimal String(number=w294) -> (decimal integer string=w293:string[])  [unwired: 1 in]
              n175 = Build Array (concatenate)(w292, w293) -> (w291:string[])
            }
            n176 = property on="Wheels" class="MCListbox (strict)"("ItemNames"=w286, "Val(Sgnl)"=0 ("Wheels")) -> ()  [unwired: 2 in, 2 out]
          }
          frame "Show Filter Wheels" {
            (unwired) string[] ["Grism", "blocked", "VPH", "open", "J", "Y"] ("Array")
            n177 = Unbundle By Name(w300) -> ("Filter Wheel Info.Filters"=w299:T8[], "FW refs"=w298:refnum<vi>[])
            n178 = for {
              tunnel: w299 -> [w311] mode=indexing
              tunnel: w298 -> [w310] mode=indexing
              tunnel: [w305] -> w297 mode=indexing
              w301 = TRUE ("Visible")
              n179 = Unbundle By Name(w311) -> ("Wheel Name"=w307:string, "Names"=w302:string[])
              n180 = control-ref of="Gauge 0"() -> (w308:refnum<vi>)
              n181 = To More Specific Class(target class=w308, reference=w310) -> (specific class reference=w309:refnum<vi>)  [unwired: 1 in, 1 out]
              n182 = property class="Knob (strict)"(reference=w309, "Visible"=w301, "TextLbls[]"=w302, "Caption.Text"=w307, "Visible"=w301) -> (error out=w303:errorcluster)  [unwired: 1 in, 1 out]
              n183 = Array Size(array=w302) -> (size(s)=w306:i32)
              n184 = Number To Decimal String(number=w306) -> (decimal integer string=w304:string)  [unwired: 1 in]
              n185 = Build Array(w307, w304) -> (w305:string[])
              n186 = call <vilib>:"Clear Errors.vi"("error in (no error)"=w303) -> ()  [unwired: 5 in, 2 out]
            }
            n187 = property on="Wheels" class="MCListbox (strict)"("ItemNames"=w297) -> ()  [unwired: 2 in, 2 out]
          }
          frame "show command" {
            n188 = Unbundle By Name(w313) -> ("Motor #"=w312:u8)
            n189 = call "Arduino Generate Command String.vi"("Filter Wheel Settings"="Filter Wheel Settings", "MOTOR NUMBER"=w312) -> ("Cmd String"=w315:string)  [unwired: 9 in]
            n190 = property on="Command Preview" class="Str"("Value"=w315) -> ()  [unwired: 2 in, 2 out]
          }
          frame "Command" {
            n191 = Unbundle By Name(w322) -> ("state"=w324:refnum<user-event>, "Data Q"=w325:refnum<queue>, "Cmd.Cmd"=w320:string, "Cmd.Parameters"=w318:variant)
            n192 = Variant To Flattened String(Variant=w318) -> (data string=w319:string)  [unwired: 1 out]
            n193 = Format Into String(format string="Filter Wheel Command %s. Parameters %s" ("Message"), w320, w319) -> (resulting string=w317:string)  [unwired: 2 in, 1 out]
            n194 = call "CC System Message.vi"("Message"=w317) -> ("error out"=w316:errorcluster)  [unwired: 10 in]
            n195 = case shown="\"Move\"" w320 {
              selector: w320 -> [w335 _ _ _ _ _]
              tunnel: w325 -> [w340 _ _ _ _ _]
              tunnel: w318 -> [_ w350 w354 _ _ _]
              tunnel: w324 -> [w329 w346 _ w357 w359 w363]
              tunnel: w322 -> [w333 w341 w351 w355 w358 w361]
              tunnel: [w327 w347 w351 w355 w358 w361] -> w323
              tunnel: w316 -> [_ _ _ _ _ _]
              frame "False", Default {
                n196 = Generate User Event(user event=w329, event data cluster="Error" ("event data")) -> ()  [unwired: 2 in, 2 out]
                n197 = Format Into String(format string="Filter Wheel received invalid command. Cmd: %s", w335) -> (resulting string=w332:string)  [unwired: 2 in, 1 out]
                n198 = call "lib Quick Message Log.vi"("Message"=w335) -> ("Log"=→"Messages":string)  [unwired: 9 in, 1 out]
                n199 = Bundle By Name(cluster=T16 {"Source"="", "Type"="", "Data"=variant} ("element"), "Source"="Message" ("Data Type"), "Data"=w332) -> (w336:T16)
                n200 = Bundle By Name(cluster=w333, "Error State"="Command", "error.status"=TRUE, "error.code"=5000, "error.source"=w332) -> (w327:T13)
                n201 = Enqueue Element(queue=w340, element=w336) -> ()  [unwired: 2 in, 3 out]
              }
              frame "Move" {
                n202 = Generate User Event(user event=w346, event data cluster="Move" ("event data")) -> ()  [unwired: 2 in, 2 out]
                n203 = Get Date/Time In Seconds() -> (seconds since 1Jan1904=w343:timestamp)
                n204 = Bundle By Name(cluster=w341, "Period"=1.0, "next poll"=w343) -> (w342:T13)
                n205 = Variant To Data(type=T9 {"Wheel ID"=0, "Position"=0}, Variant=w350) -> (data=w348:T9)  [unwired: 1 in, 1 out]
                n206 = Bundle By Name(cluster=w342, "Move"=w348) -> (w347:T13)
              }
              frame "MoveFilter" {
                n207 = Variant To Data(type=T17 {"Position Names"=[]}, Variant=w354) -> (data=w352:T17)  [unwired: 1 in, 1 out]
                n208 = Unbundle By Name(w352) -> ()  [unwired: 1 out]
              }
              frame "Status" {
                n209 = Generate User Event(user event=w357, event data cluster="Send Status" ("event data")) -> ()  [unwired: 2 in, 2 out]
              }
              frame "Config" {
                n210 = Generate User Event(user event=w359, event data cluster="Send Config" ("event data")) -> ()  [unwired: 2 in, 2 out]
              }
              frame "Shutdown" {
                n211 = Generate User Event(user event=w363, event data cluster="Shutdown" ("event data")) -> ()  [unwired: 2 in, 2 out]
              }
            }
          }
          frame "Move" {
            w371 = TRUE ("Visible")
            n212 = Unbundle By Name(w364) -> ("state"=w374:refnum<user-event>, "Filter Wheel ref"=w369:refnum<class "Filter Wheel.lvclass">, "Move"=w380:T9, "Filter Wheel Info"=w379:T7)
            n213 = property on="Tab Control" class="TabCtl (strict)"() -> ("Pages"=w378:refnum<vi>[])  [unwired: 2 in, 2 out]
            n214 = Index Array(array=w378, index=0) -> (element=w376:refnum<vi>)
            n215 = Get Date/Time In Seconds() -> (seconds since 1Jan1904=w366:timestamp)
            n216 = property class="Page"(reference=w376, "PageEnb"=T18."Page Disabled & Grayed" ("Page Enabled State")) -> ()  [unwired: 1 in, 2 out]
            n217 = Bundle By Name(cluster=w364, "Period"=1.0, "next poll"=w366) -> (w365:T13)
            n218 = call "Filter Wheel Validate Move Command.vi"("Filter Wheel Info"=w379, "Move"=w380) -> ("error out"=w370:errorcluster, "Move dup"=w368:T9)  [unwired: 7 in, 1 out]
            n219 = case shown="No Error" w370 {
              selector: w370 -> [_ w398]
              tunnel: w374 -> [w396 w404]
              tunnel: w365 -> [w391 w402]
              tunnel: [w392 w401] -> w373
              tunnel: [w382 w399] -> w372
              tunnel: w369 -> [w395 _]
              tunnel: w368 -> [w394 _]
              frame No Error {
                n220 = Unbundle By Name(w394) -> ("Wheel ID"=w384:i32, "Position"=w383:i32)
                n221 = call-dynamic "Write Wheel Run State.vi"("Run"=TRUE, "Wheel"=w384, "Filter Wheel in"=w395) -> ("Filter Wheel out"=w387:refnum<class "Filter Wheel.lvclass">)  [unwired: 7 in, 1 out]
                n222 = Generate User Event(user event=w396, event data cluster="send data" ("event data")) -> (user event out=w389:refnum<user-event>)  [unwired: 2 in, 1 out]
                n223 = call-dynamic "Get Status.vi"("Filter Wheel in"=w387) -> ("FW Status"=w381:T11, "Filter Wheel out"=w386:refnum<class "Filter Wheel.lvclass">)  [unwired: 8 in, 1 out]
                n224 = Generate User Event(user event=w389, event data cluster="Move Finish" ("event data")) -> ()  [unwired: 2 in, 2 out]
                n225 = Bundle By Name(cluster=w391, "Filter Wheel ref"=w386, "FW Status"=w381) -> (w392:T13)
                n226 = Format Into String(format string="Initiating filter wheel %d move to position %d.", w384, w383) -> (resulting string=w382:string)  [unwired: 2 in, 1 out]
              }
              frame Error {
                n227 = Generate User Event(user event=w404, event data cluster="Error" ("event data")) -> ()  [unwired: 2 in, 2 out]
                n228 = Unbundle By Name(w398) -> ("source"=w397:string)
                n229 = Format Into String(format string="Filter Wheel Move Error: %s", w397) -> (resulting string=w399:string)  [unwired: 2 in, 1 out]
                n230 = Bundle By Name(cluster=w402, "error"=w398, "Error State"=w399) -> (w401:T13)
              }
            }
            n231 = property on="Moving Message" class="Str"("Visible"=w371, "Blinking"=w371) -> ()  [unwired: 2 in, 2 out]
            n232 = call "CC System Message.vi"("Message"=w372) -> ()  [unwired: 10 in, 1 out]
          }
          frame "Move Finish" {
            w417 = FALSE ("Visible")
            n233 = Unbundle By Name(w422) -> ("state"=w424:refnum<user-event>, "Filter Wheel ref"=w427:refnum<class "Filter Wheel.lvclass">, "Move"=w416:T9)
            n234 = property on="Tab Control" class="TabCtl (strict)"() -> ("Pages"=w415:refnum<vi>[])  [unwired: 2 in, 2 out]
            n235 = local read "Last Move Positions"() -> (w408:u32[])
            n236 = Unbundle By Name(w416) -> ("Wheel ID"=w406:i32, "Position"=w425:i32)
            n237 = Index Array(array=w415, index=0) -> (element=w413:refnum<vi>)
            n238 = call-dynamic "Set One Filter.vi"("Position (0:4)"=w425, "Filter Wheel (0:n-1)"=w406, "Filter Wheel in"=w427) -> ("error out"=w409:errorcluster, "Target Counts"=w405:i32, "Filter Wheel out"=w412:refnum<class "Filter Wheel.lvclass">, "Message"=w420:string)  [unwired: 3 in, 2 out]
            n239 = Replace Array Subset(array=w408, new element=w405, index=w406) -> (→"Last Move Positions":u32[])
            n240 = call-dynamic "Write Wheel Run State.vi"("Run"=FALSE, "Wheel"=w406, "Filter Wheel in"=w412) -> ("Filter Wheel out"=w410:refnum<class "Filter Wheel.lvclass">)  [unwired: 7 in, 1 out]
            n241 = case shown="Error .." w409 {
              selector: w409 -> [_ w441]
              tunnel: w424 -> [_ w444]
              tunnel: w422 -> [w433 w442]
              tunnel: [w431 w440] -> w423
              tunnel: w413 -> [w434 w439]
              tunnel: [w434 w439] -> w421
              tunnel: w410 -> [w432 w435]
              tunnel: w420 -> [w429 w437]
              tunnel: ["Move complete." ("string") w436] -> w419
              frame No Error {
                n242 = call "CC System Message.vi"("Message"=w429) -> ()  [unwired: 10 in, 1 out]
                n243 = Bundle By Name(cluster=w433, "Filter Wheel ref"=w432, "Period"=30.0) -> (w431:T13)
              }
              frame Error {
                n244 = Generate User Event(user event=w444, event data cluster="Error" ("event data")) -> ()  [unwired: 2 in, 2 out]
                n245 = Format Into String(format string="Filter Wheel Move Error: %s", w437) -> (resulting string=w436:string)  [unwired: 2 in, 1 out]
                n246 = Bundle By Name(cluster=w442, "Filter Wheel ref"=w435, "error"=w441, "Error State"=w436) -> (w440:T13)
              }
            }
            n247 = property class="Page"(reference=w421, "PageEnb"=T18."Page Enabled" ("Page Enabled State")) -> (error out=w418:errorcluster)  [unwired: 1 in, 1 out]
            n248 = property on="Moving Message" class="Str"(error in=w418, "Visible"=w417, "Blinking"=w417) -> ()  [unwired: 1 in, 2 out]
            n249 = call "CC System Message.vi"("Message"=w419) -> ()  [unwired: 10 in, 1 out]
          }
          frame "Home" {
            w462 = TRUE ("Visible")
            n250 = property on="Moving Message" class="Str"("Visible"=w462, "Blinking"=w462) -> (error out=w461:errorcluster)  [unwired: 2 in, 1 out]
            n251 = Unbundle By Name(w445) -> ("state"=w456:refnum<user-event>, "Filter Wheel ref"=w460:refnum<class "Filter Wheel.lvclass">)
            n252 = Format Into String(format string="Home started on wheel %d", "Wheel To Home") -> (resulting string=w464:string)  [unwired: 2 in, 1 out]
            n253 = call "CC System Message.vi"("error in (no error)"=w461, "Message"=w464) -> ("error out"=w457:errorcluster)  [unwired: 9 in]
            n254 = Get Date/Time In Seconds() -> (seconds since 1Jan1904=w447:timestamp)
            n255 = call-dynamic "Write Wheel Run State.vi"("error in (no error)"=w457, "Run"=TRUE, "Wheel"="Wheel To Home", "Filter Wheel in"=w460) -> ("error out"=w449:errorcluster, "Filter Wheel out"=w452:refnum<class "Filter Wheel.lvclass">)  [unwired: 6 in]
            n256 = Generate User Event(user event=w456, event data cluster="send data" ("event data")) -> (user event out=w455:refnum<user-event>)  [unwired: 2 in, 1 out]
            n257 = Bundle By Name(cluster=w445, "Period"=1.0, "next poll"=w447) -> (w446:T13)
            n258 = call-dynamic "Get Status.vi"("error in (no error)"=w449, "Filter Wheel in"=w452) -> ("FW Status"=w450:T11, "Filter Wheel out"=w451:refnum<class "Filter Wheel.lvclass">)  [unwired: 7 in, 1 out]
            n259 = Generate User Event(user event=w455, event data cluster="Home Finish" ("event data")) -> ()  [unwired: 2 in, 2 out]
            n260 = Bundle By Name(cluster=w446, "Filter Wheel ref"=w451, "FW Status"=w450) -> (w463:T13)
          }
          frame "Home Finish" {
            w471 = FALSE ("Visible")
            n261 = local read "Wheel To Home"() -> (w467:u16)
            n262 = Unbundle By Name(w473) -> ("state"=w474:refnum<user-event>, "Filter Wheel ref"=w477:refnum<class "Filter Wheel.lvclass">)
            n263 = call-dynamic "Home Filter Wheel.vi"("Motor"=w467, "Filter Wheel in"=w477) -> ("error out"=w475:errorcluster, "Log"=w476:string, "Filter Wheel out"=w469:refnum<class "Filter Wheel.lvclass">)  [unwired: 6 in, 1 out]
            n264 = call "CC System Message.vi"("Message"=w476) -> ("error out"=w470:errorcluster)  [unwired: 10 in]
            n265 = call-dynamic "Write Wheel Run State.vi"("Run"=FALSE, "Wheel"=w467, "Filter Wheel in"=w469) -> ("Filter Wheel out"=w468:refnum<class "Filter Wheel.lvclass">)  [unwired: 7 in, 1 out]
            n266 = case shown="Error .." w475 {
              selector: w475 -> [_ w486]
              tunnel: w474 -> [_ w484]
              tunnel: w473 -> [w479 w487]
              tunnel: [w480 w485] -> w472
              tunnel: w468 -> [w481 _]
              frame No Error {
                n267 = Bundle By Name(cluster=w479, "Filter Wheel ref"=w481, "Period"=30.0) -> (w480:T13)
              }
              frame Error {
                n268 = Generate User Event(user event=w484, event data cluster="Error" ("event data")) -> ()  [unwired: 2 in, 2 out]
                n269 = Bundle By Name(cluster=w487, "error"=w486, "Error State"="Homing") -> (w485:T13)
              }
            }
            n270 = property on="Moving Message" class="Str"(error in=w470, "Visible"=w471, "Blinking"=w471) -> ()  [unwired: 1 in, 2 out]
          }
          frame "Stop" {
            n271 = Unbundle By Name(w489) -> ("Filter Wheel ref"=w493:refnum<class "Filter Wheel.lvclass">)
            n272 = call-dynamic "Emergency Stop.vi"("Wheel (-1: all)"=-1, "Filter Wheel in"=w493) -> ("Filter Wheel out"=w491:refnum<class "Filter Wheel.lvclass">)  [unwired: 8 in, 1 out]
            n273 = Bundle By Name(cluster=w489, "Filter Wheel ref"=w491) -> (w490:T13)
            n274 = call "CC System Message.vi"("Message"="Filter Wheel stopped by user.") -> ()  [unwired: 10 in, 1 out]
          }
          frame "Poll" {
            # "Request status from hardware"
            n275 = Unbundle By Name(w502) -> ("state"=w501:refnum<user-event>, "Filter Wheel ref"=w496:refnum<class "Filter Wheel.lvclass">)
            n276 = property on="Filter Wheel Displays" class="Clust (strict)"() -> ("Controls[]"=w507:refnum<vi>[])  [unwired: 2 in, 2 out]
            n277 = call-dynamic "Get Status.vi"("Filter Wheel in"=w496) -> ("error out"=w498:errorcluster, "FW Status"=w495:T11, "Filter Wheel out"=w499:refnum<class "Filter Wheel.lvclass">)  [unwired: 8 in]
            n278 = call-dynamic "Read Home State.vi"("Filter Wheel in"=w496) -> ("Home State"=→"Homed":bool[])  [unwired: 8 in, 2 out]
            n279 = Generate User Event(user event=w501, event data cluster="send data" ("event data")) -> ()  [unwired: 2 in, 2 out]
            n280 = Split 1D Array(array=w507, index=8) -> (first subarray=w504:refnum<vi>[], second subarray=w505:refnum<vi>[])
            n281 = Unbundle By Name(w495) -> ("Notch"=→"On the notch":bool[])
            n282 = case shown="No Error" w498 {
              tunnel: w505 -> [w512 _]
              tunnel: w504 -> [w511 _]
              tunnel: w495 -> [w509 _]
              frame No Error {
                n283 = Unbundle By Name(w509) -> ("Positions"=w508:i32[], "Notch"=w510:bool[])
                n284 = call "Filter Wheel Update Status.vi"("FW Status"=w509) -> ()  [unwired: 10 in, 1 out]
                n285 = for {
                  tunnel: w510 -> [w514] mode=indexing
                  tunnel: w508 -> [w515] mode=indexing
                  tunnel: w512 -> [w517] mode=indexing
                  tunnel: w511 -> [w516] mode=indexing
                  n286 = Not(x=w514) -> ()  [unwired: 1 out]
                  n287 = property class="Ctl"(reference=w517, "Value"=w515) -> ()  [unwired: 1 in, 2 out]
                  n288 = property class="Ctl"(reference=w516, "Blinking"=FALSE, "Value"=w515) -> ()  [unwired: 1 in, 2 out]
                }
              }
              frame Error {
              }
            }
            n289 = Bundle By Name(cluster=w502, "Filter Wheel ref"=w499, "FW Status"=w495) -> (w503:T13)
          }
          frame "send raw string" {
            n290 = Unbundle By Name(w518) -> ("Filter Wheel ref"=w522:refnum<class "Filter Wheel.lvclass">)
            n291 = call-dynamic "Send Raw String.vi"("Cmd String"="Command Preview", "Filter Wheel in"=w522) -> ("Filter Wheel out"=w520:refnum<class "Filter Wheel.lvclass">)  [unwired: 8 in, 1 out]
            n292 = Bundle By Name(cluster=w518, "Filter Wheel ref"=w520) -> (w519:T13)
          }
          frame "read raw" {
            n293 = Unbundle By Name(w526) -> ("Filter Wheel ref"=w525:refnum<class "Filter Wheel.lvclass">)
            n294 = call-dynamic "Read Raw String.vi"("Filter Wheel in"=w525) -> ("Raw String"=→"Response":string, "Filter Wheel out"=w524:refnum<class "Filter Wheel.lvclass">)  [unwired: 8 in, 1 out]
            n295 = Bundle By Name(cluster=w526, "Filter Wheel ref"=w524) -> (w527:T13)
          }
          frame "Send Config" {
            n296 = Unbundle By Name(w533) -> ("Data Q"=w532:refnum<queue>, "Filter Wheel Info"=w529:T7)
            n297 = Bundle By Name(cluster=T16 {"Source"="", "Type"="", "Data"=variant} ("element"), "Source"="Filter Wheel Config" ("Data Type"), "Data"=w529) -> (w528:T16)
            n298 = Enqueue Element(queue=w532, element=w528) -> ()  [unwired: 2 in, 3 out]
          }
          frame "Send Status" {
            n299 = Unbundle By Name(w540) -> ("Data Q"=w539:refnum<queue>, "Filter Wheel ref"=w535:refnum<class "Filter Wheel.lvclass">)
            n300 = call-dynamic "Get Status.vi"("Filter Wheel in"=w535) -> ("FW Status"=w534:T11)  [unwired: 8 in, 2 out]
            n301 = Bundle By Name(cluster=T16 {"Source"="", "Type"="", "Data"=variant} ("element"), "Source"="Filter Wheel Status" ("Data Type"), "Data"=w534) -> (w536:T16)
            n302 = Enqueue Element(queue=w539, element=w536) -> ()  [unwired: 2 in, 3 out]
          }
          frame "Error" {
            w547 = "Filter Wheel" ("Source")
            n303 = Unbundle By Name(w545) -> ("error.status"=w554:bool, "Data Q"=w550:refnum<queue>, "Error State"=w542:string)
            n304 = Bundle By Name(cluster=T19 {"Measured Value"=0.0, "Alarm Low"=0.0, "Alarm High"=0.0, "Message"="", "Source"=""} ("element"), "Source"=w547, "Message"=w542) -> (w548:T19)
            n305 = property on="Error" class="Bool (strict)"("Value"=w554) -> ()  [unwired: 2 in, 2 out]
            n306 = Bundle By Name(cluster=T16 {"Source"="", "Type"="", "Data"=variant} ("element"), "Source"=w547, "Type"="Alarm Set", "Data"=w548) -> (w551:T16)
            n307 = Format Into String(format string="Filter Wheel Error: %s", w542) -> (resulting string=w541:string)  [unwired: 2 in, 1 out]
            n308 = Enqueue Element(queue=w550, element=w551) -> ()  [unwired: 2 in, 3 out]
            n309 = Bundle By Name(cluster=w545, "Period"=30.0) -> (w546:T13)
            n310 = call "CC System Message.vi"("Message"=w541) -> ()  [unwired: 10 in, 1 out]
          }
          frame "Ready" {
            w558 = "Filter Wheel" ("Source")
            n311 = Unbundle By Name(w566) -> ("Data Q"=w562:refnum<queue>, "Error State"=w559:string)
            n312 = Bundle By Name(cluster=T19 {"Measured Value"=0.0, "Alarm Low"=0.0, "Alarm High"=0.0, "Message"="", "Source"=""} ("element"), "Source"=w558, "Message"=w559) -> (w560:T19)
            n313 = Bundle By Name(cluster=T16 {"Source"="", "Type"="", "Data"=variant} ("element"), "Source"=w558, "Type"="Alarm Clear", "Data"=w560) -> (w563:T16)
            n314 = Enqueue Element(queue=w562, element=w563) -> (error out=w556:errorcluster)  [unwired: 2 in, 2 out]
            n315 = call "CC System Message.vi"("Message"="Filter Wheel Ready") -> ()  [unwired: 10 in, 1 out]
            n316 = property on="Error" class="Bool (strict)"(error in=w556, "Value"=FALSE ("Error")) -> ()  [unwired: 1 in, 2 out]
          }
          frame "Shutdown" {
            n317 = Unbundle By Name(w569) -> ("Filter Wheel ref"=w568:refnum<class "Filter Wheel.lvclass">)
            n318 = call-dynamic "Close.vi"("Filter Wheel in"=w568) -> ()  [unwired: 9 in, 2 out]
            n319 = call "CC System Message.vi"("Message"="Filter Wheel shutdown.") -> ()  [unwired: 10 in, 1 out]
          }
        }
      }
      event "Standalone": Value Change {
        n320 = event-data() -> ("NewVal"=w571:bool)  [unwired: 1 in]
        n321 = property on="Close" class="Bool"("Visible"=w571) -> ()  [unwired: 2 in, 2 out]
      }
      event "Alarms?": Value Change {
        n322 = event-data() -> ()  [unwired: 1 in, 6 out]
        n323 = Unbundle By Name(w574) -> ("Filter Wheel ref"=w577:refnum<class "Filter Wheel.lvclass">)
        n324 = property class="Filter Wheel.lvclass"(reference=w577, "Alarms_"="Alarms?") -> (reference out=w575:refnum<class "Filter Wheel.lvclass">)  [unwired: 1 in, 1 out]
        n325 = Bundle By Name(cluster=w574, "Filter Wheel ref"=w575) -> (w573:T13)
      }
      event "Open Arduino Log": Value Change {
        n326 = event-data() -> ()  [unwired: 1 in, 6 out]
        n327 = Unbundle By Name(w583) -> ()  [unwired: 1 out]
        n328 = call <vilib>:"Dflt Data Dir.vi"() -> ("App:Default Data Directory"=w582:path)
        n329 = Build Path(base path=w582, name or relative path="Logs") -> (appended path=w580:path)
        n330 = Build Path(base path=w580, name or relative path="Filter Wheel") -> (appended path=w578:path)
        n331 = call <vilib>:"Show in File System.vi"("file or directory path"=w578) -> ()  [unwired: 10 in, 1 out]
      }
      event "Filter Wheel Table": Value Change {
        n332 = event-data() -> ()  [unwired: 1 in, 6 out]
        n333 = call "Rd Wr settings json Filter Wheel Table.vi"("Write? (F:Read)"=TRUE, "Filter Wheel Table"="Filter Wheel Table") -> ()  [unwired: 8 in, 2 out]
      }
      event "Read": Value Change {
        n334 = event-data() -> ()  [unwired: 1 in, 6 out]
        n335 = Unbundle By Name(w589) -> ("state"=w588:refnum<user-event>)
        n336 = Generate User Event(user event=w588, event data cluster="read raw" ("event data")) -> ()  [unwired: 2 in, 2 out]
      }
      event "Error": Value Change {
        n337 = event-data() -> ()  [unwired: 1 in, 6 out]
        n338 = Unbundle By Name(w591) -> ("Error State"=w592:string, "error.code"=w599:i32, "error.source"=w598:string, "error.status"=w597:bool)
        n339 = Format Into String(format string="An error occurred during %s. \nError Number: %d\nError message: %s", w592, w599, w598) -> (resulting string=w596:string)  [unwired: 2 in, 1 out]
        n340 = call "Display Message to User"("Enable"=w597, "Message"=w596) -> ("error out"=w593:errorcluster, "Close"=w595:bool)  [unwired: 8 in]
        n341 = Unbundle By Name(w591) -> ("state"=w590:refnum<user-event>)
        n342 = case shown="True" w595 {
          selector: w595 -> [w601 _]
          tunnel: w591 -> [w604 w607]
          tunnel: [w602 w607] -> w594
          tunnel: w593 -> [w603 _]
          tunnel: w590 -> [_ w606]
          frame False {
            n343 = property on="Error" class="Bool (strict)"("Value"=w601) -> ()  [unwired: 2 in, 2 out]
            n344 = Bundle By Name(cluster=w604, "error"=w603) -> (w602:T13)
          }
          frame True {
            n345 = Generate User Event(user event=w606, event data cluster="Ready" ("event data")) -> ()  [unwired: 2 in, 2 out]
          }
        }
      }
      event Value Change {
        n346 = event-data() -> ()  [unwired: 1 in, 6 out]
        n347 = Unbundle By Name(w613) -> ("Filter Wheel ref"=w616:refnum<class "Filter Wheel.lvclass">, "Name"=w608:string)
        n348 = call "Rd Wr Filter Wheel Settings.vi"("Wheel Name"=w608) -> ("Filter Wheel Settings"=w612:T7)  [unwired: 9 in, 1 out]
        n349 = call-dynamic "Write Homing.vi"("Homing"="Movement Parameters", "Filter Wheel in"=w616) -> ("Filter Wheel out"=w615:refnum<class "Filter Wheel.lvclass">)  [unwired: 8 in, 1 out]
        n350 = Bundle By Name(cluster=w612, "Homing Parameters"="Movement Parameters") -> (w610:T7)
        n351 = Bundle By Name(cluster=w613, "Filter Wheel ref"=w615) -> (w614:T13)
        n352 = call "Rd Wr Filter Wheel Settings.vi"("Wheel Name"=w608, "Write? (F:Read)"=TRUE, "Filter Wheel Settings"=w610) -> ()  [unwired: 7 in, 2 out]
      }
      event "Default Speed": Value Change {
        n353 = event-data() -> ()  [unwired: 1 in, 6 out]
        n354 = Unbundle By Name(w620) -> ("Filter Wheel ref"=w626:refnum<class "Filter Wheel.lvclass">, "Name"=w617:string)
        n355 = call-dynamic "Read Filter Wheel Info.vi"("Filter Wheel in"=w626) -> ("Filter Wheel Info"=w624:T7, "Filter Wheel out"=w625:refnum<class "Filter Wheel.lvclass">)  [unwired: 8 in, 1 out]
        n356 = Bundle By Name(cluster=w624, "Default Speed"="Default Speed") -> (w618:T7)
        n357 = call-dynamic "Write Filter Wheel Info.vi"("Filter Wheel Info"=w618, "Filter Wheel in"=w625) -> ("Filter Wheel out"=w622:refnum<class "Filter Wheel.lvclass">)  [unwired: 8 in, 1 out]
        n358 = call "Rd Wr Filter Wheel Settings.vi"("Wheel Name"=w617, "Write? (F:Read)"=TRUE, "Filter Wheel Settings"=w618) -> ()  [unwired: 7 in, 2 out]
        n359 = Bundle By Name(cluster=w620, "Filter Wheel ref"=w622) -> (w621:T13)
      }
      event "Home": Value Change {
        n360 = event-data() -> ()  [unwired: 1 in, 6 out]
        n361 = Unbundle By Name(w629) -> ("state"=w628:refnum<user-event>)
        n362 = Generate User Event(user event=w628, event data cluster="Home" ("event data")) -> ()  [unwired: 2 in, 2 out]
      }
      event "Simulate": Value Change {
        n363 = event-data() -> ()  [unwired: 1 in, 6 out]
        n364 = Unbundle By Name(w635) -> ("state"=w634:refnum<user-event>)
        n365 = Select(t="set simulation on" ("event data"), s="Simulate", f="set simulation off" ("event data")) -> (s? t:f=w631:string)
        n366 = Generate User Event(user event=w634, event data cluster=w631) -> ()  [unwired: 2 in, 2 out]
      }
      event "Sim Velocity (steps/sec)": Value Change {
        n367 = event-data() -> ()  [unwired: 1 in, 6 out]
        n368 = Unbundle By Name(w636) -> ("Simulate"=w639:bool, "Filter Wheel ref"=w640:refnum<class "Filter Wheel.lvclass">)
        n369 = case shown="True" w639 {
          tunnel: w640 -> [_ w648]
          tunnel: "Sim Velocity (steps/sec)" -> [_ w645]
          tunnel: w636 -> [w641 w644]
          tunnel: [w641 w642] -> w637
          frame False {
          }
          frame True {
            n370 = To More Specific Class(target class=refnum<class "Filter Wheel Simulator.lvclass"> refnum ("Filter Wheel Simulator.lvclass"), reference=w648) -> (specific class reference=w646:refnum<class "Filter Wheel Simulator.lvclass">)  [unwired: 1 in, 1 out]
            n371 = call "Write Velocity (cnts_sec).vi"("Velocity (cnts/sec)"=w645, "Filter Wheel Simulator in"=w646) -> ("Filter Wheel Simulator out"=w643:refnum<class "Filter Wheel Simulator.lvclass">)  [unwired: 8 in, 1 out]
            n372 = Bundle By Name(cluster=w644, "Filter Wheel ref"=w643) -> (w642:T13)
          }
        }
      }
      event "Connect": Value Change {
        n373 = event-data() -> ()  [unwired: 1 in, 6 out]
        n374 = Unbundle By Name(w651) -> ("state"=w650:refnum<user-event>)
        n375 = Generate User Event(user event=w650, event data cluster="connect" ("event data")) -> ()  [unwired: 2 in, 2 out]
      }
      event Value Change {
        n376 = event-data() -> ()  [unwired: 1 in, 1 out]
        n377 = Unbundle By Name(w654) -> ("state"=w653:refnum<user-event>)
        n378 = Generate User Event(user event=w653, event data cluster="show command" ("event data")) -> ()  [unwired: 2 in, 2 out]
      }
      event "Send Command": Value Change {
        n379 = event-data() -> ()  [unwired: 1 in, 6 out]
        n380 = Unbundle By Name(w657) -> ("state"=w656:refnum<user-event>)
        n381 = Generate User Event(user event=w656, event data cluster="send raw string" ("event data")) -> ()  [unwired: 2 in, 2 out]
      }
      event "MOTOR NUMBER": Value Change {
        n382 = event-data() -> ("NewVal"=w660:u8)  [unwired: 1 in]
        n383 = Bundle By Name(cluster=w658, "Motor #"=w660) -> (w659:T13)
      }
      event "STOP": Value Change {
        n384 = event-data() -> ()  [unwired: 1 in, 6 out]
        n385 = Unbundle By Name(w663) -> ("state"=w662:refnum<user-event>)
        n386 = Generate User Event(user event=w662, event data cluster="Stop" ("event data")) -> ()  [unwired: 2 in, 2 out]
      }
      event Value Change {
        n387 = event-data() -> ()  [unwired: 1 in, 1 out]
        n388 = Unbundle By Name(w666) -> ("state"=w665:refnum<user-event>)
        n389 = Generate User Event(user event=w665, event data cluster="set mode" ("event data")) -> ()  [unwired: 2 in, 2 out]
      }
      event "Filter Wheel Displays": Value Change {
        n390 = event-data() -> ("OldVal"=w674:T3, "NewVal"=w667:T3)  [unwired: 1 in]
        n391 = Unbundle By Name(w675) -> ("state"=w678:refnum<user-event>)
        n392 = Not Equal?(x=w674, y=w667) -> (x != y?=w673:T21)
        n393 = Cluster To Array(cluster=w667) -> (array=w670:i32[])
        n394 = Cluster To Array(cluster=w673) -> (array=w672:bool[])
        n395 = Generate User Event(user event=w678, event data cluster="Move" ("event data")) -> ()  [unwired: 2 in, 2 out]
        n396 = Search 1D Array(1D array=w672, element=TRUE) -> (index of element=w668:i32)  [unwired: 1 in]
        n397 = Index Array(array=w670, index=w668) -> (element=w669:i32)
        n398 = Bundle By Name(cluster=w675, "Move.Wheel ID"=w668, "Move.Position"=w669) -> (w676:T13)
      }
      event "Wheels": Value Change {
        n399 = event-data() -> ("NewVal"=w681:i32)  [unwired: 1 in]
        n400 = Unbundle By Name(w679) -> ("Pos Names"=w684:cluster{"Table":string[][]}[])
        n401 = Index Array(array=w684, index=w681) -> (element=w683:cluster{"Table":string[][]})
        n402 = Unbundle(w683) -> ("Table"=w682:string[][])
        n403 = property on="Positions" class="MCListbox (strict)"("ItemNames"=w682) -> ()  [unwired: 2 in, 2 out]
        n404 = Bundle By Name(cluster=w679, "Wheel"=w681) -> (w680:T13)
      }
      event "Wheels": Edit Cell? {
        n405 = event-data() -> ("String"=w688:string, "Coords"=w687:T10)  [unwired: 1 in]
        n406 = Unbundle By Name(w687) -> ("Column"=w690:i32)
        n407 = Not Equal To 0?(x=w690) -> (x != 0?=w689:bool)
        n408 = Bundle By Name(cluster=w685, "Coords"=w687) -> (w686:T13)
        n409 = event-data("String"=w688, "Discard?"=w689) -> ()  [unwired: 1 in, 1 out]
      }
      event "Wheels": Edit Cell {
        n410 = event-data() -> ("String"=w695:string)  [unwired: 1 in]
        n411 = Unbundle By Name(w692) -> ("FW names"=w696:string[], "Coords.Row"=w691:i32)
        n412 = Replace Array Subset(array=w696, new element=w695, index=w691) -> (w694:string[])
        n413 = Bundle By Name(cluster=w692, "FW names"=w694) -> (w693:T13)
      }
      event "Positions": Edit Cell? {
        n414 = event-data() -> ("String"=w702:string, "Coords"=w699:T10)  [unwired: 1 in, 4 out]
        n415 = Unbundle By Name(w699) -> ("Column"=w703:i32)
        n416 = case shown="0, Default" w703 {
          tunnel: w702 -> [w705 w711]
          tunnel: [w705 w708] -> w701
          tunnel: [FALSE ("status") w706] -> w700
          frame 0, Default {
          }
          frame 1 {
            w710 = "%d" ("format string")
            n417 = Scan From String(format string=w710, input string=w711) -> (error out=w707:errorcluster, output 1=w709:i32)  [unwired: 3 in, 2 out]
            n418 = Unbundle By Name(w707) -> ("status"=w706:bool)
            n419 = Format Into String(format string=w710, w709) -> (resulting string=w708:string)  [unwired: 2 in, 1 out]
          }
        }
        n420 = Bundle By Name(cluster=w697, "Coords"=w699) -> (w698:T13)
        n421 = event-data("String"=w701, "Discard?"=w700) -> ()  [unwired: 1 in, 1 out]
      }
      event "Positions": Edit Cell {
        n422 = event-data() -> ("String"=w720:string)  [unwired: 1 in, 5 out]
        n423 = Unbundle By Name(w713) -> ("Pos Names"=w718:cluster{"Table":string[][]}[], "Coords"=w712:T10)
        n424 = Unbundle By Name(w712) -> ("Row"=w721:i32, "Column"=w722:i32)
        n425 = Index Array(array=w718, index="Wheels") -> (element=w724:cluster{"Table":string[][]})
        n426 = Unbundle(w724) -> ("Table"=w723:string[][])
        n427 = Replace Array Subset(array=w723, new element=w720, index (row)=w721, index (col)=w722) -> (w719:string[][])
        n428 = Bundle("Table"=w719) -> (w717:cluster{"Table":string[][]})  [unwired: 1 in]
        n429 = Replace Array Subset(array=w718, new element=w717, index="Wheels") -> (w715:cluster{"Table":string[][]}[])
        n430 = Bundle By Name(cluster=w713, "Pos Names"=w715) -> (w714:T13)
      }
      event "Add Pos": Value Change {
        n431 = event-data() -> ()  [unwired: 1 in, 6 out]
        n432 = Unbundle By Name(w735) -> ("Pos Names"=w731:cluster{"Table":string[][]}[], "Wheel"=w730:i32)  [unwired: 1 out]
        n433 = Index Array(array=w731, index=w730) -> (element=w729:cluster{"Table":string[][]})
        n434 = Build Array("Unnamed", "0") -> (w732:string[])
        n435 = Unbundle By Name(w729) -> ("Table"=w726:string[][])
        n436 = Build Array (concatenate)(w726, w732) -> (w725:string[][])
        n437 = Bundle By Name(cluster=w729, "Table"=w725) -> (w728:cluster{"Table":string[][]})
        n438 = property on="Positions" class="MCListbox (strict)"("ItemNames"=w725) -> ()  [unwired: 2 in, 2 out]
        n439 = Replace Array Subset(array=w731, new element=w728, index=w730) -> (w727:cluster{"Table":string[][]}[])
        n440 = Bundle By Name(cluster=w735, "Pos Names"=w727) -> (w736:T13)
      }
      event "Remove Pos": Value Change {
        n441 = event-data() -> ()  [unwired: 1 in, 6 out]
        n442 = Unbundle By Name(w744) -> ("Pos Names"=w738:cluster{"Table":string[][]}[], "Wheel"=w743:i32)
        n443 = Index Array(array=w738, index=w743) -> (element=w740:cluster{"Table":string[][]})
        n444 = Unbundle By Name(w740) -> ("Table"=w742:string[][])
        n445 = Delete From Array(array=w742, index (row)="Positions") -> (array with subset deleted=w737:string[][])  [unwired: 2 in, 1 out]
        n446 = Bundle By Name(cluster=w740, "Table"=w737) -> (w739:cluster{"Table":string[][]})
        n447 = property on="Positions" class="MCListbox (strict)"("ItemNames"=w737) -> ()  [unwired: 2 in, 2 out]
        n448 = Replace Array Subset(array=w738, new element=w739, index=w743) -> (w746:cluster{"Table":string[][]}[])
        n449 = Bundle By Name(cluster=w744, "Pos Names"=w746) -> (w745:T13)
      }
      event "Add Fw": Value Change {
        n450 = event-data() -> ()  [unwired: 1 in, 6 out]
        n451 = Unbundle By Name(w750) -> ("FW names"=w748:string[], "Pos Names"=w749:cluster{"Table":string[][]}[])
        n452 = Array Size(array=w748) -> (size(s)=w747:i32)
        n453 = case shown="0..4" w747 {
          tunnel: w748 -> [_ w769]
          tunnel: [w753 w768] -> w751
          tunnel: w750 -> [w753 w767]
          tunnel: w749 -> [_ w756]
          frame 5, Default {
            n454 = One Button Dialog(message="Maximum of 4 filter wheels") -> ()  [unwired: 1 in, 1 out]
          }
          frame 0..4 {
            w760 = "Unnamed"
            n455 = Build Array (concatenate)(w756, cluster{"Table":string[][]} {"Table"=[]}) -> (w754:cluster{"Table":string[][]}[])
            n456 = property on="Wheels" class="MCListbox (strict)"() -> ("ItemNames"=w761:string[][])  [unwired: 2 in, 2 out]
            n457 = Build Array (concatenate)(w769, w760) -> (w763:string[])
            n458 = Build Array(w760, "0" ("element")) -> (w758:string[])
            n459 = Array Size(array=w763) -> (size(s)=w765:i32)
            n460 = Decrement(x=w765) -> (x-1=w764:i32)
            n461 = Build Array (concatenate)(w761, w758) -> (w757:string[][])
            n462 = property on="Wheels" class="MCListbox (strict)"("ItemNames"=w757) -> (error out=w762:errorcluster)  [unwired: 2 in, 1 out]
            n463 = Bundle By Name(cluster=T10 {"Row"=0, "Column"=0} ("Active Cell:Active Cell"), "Row"=w764) -> (w766:T10)
            n464 = Bundle By Name(cluster=w767, "Filter Wheel Info.Num Wheels"=w765, "FW names"=w763, "Pos Names"=w754) -> (w768:T13)
            n465 = property on="Wheels" class="MCListbox (strict)"(error in=w762, "ActiveCell"=w766, "FocusRow"=w764) -> ()  [unwired: 1 in, 2 out]
          }
        }
      }
      event "Remove Fw": Value Change {
        w775 = 1 ("length")
        n466 = event-data() -> ()  [unwired: 1 in, 6 out]
        n467 = Unbundle By Name(w773) -> ("FW names"=w780:string[], "Pos Names"=w779:cluster{"Table":string[][]}[], "Wheel"=w778:i32, "state"=w772:refnum<user-event>)
        n468 = Generate User Event(user event=w772, event data cluster="Show Tables" ("event data")) -> ()  [unwired: 2 in, 2 out]
        n469 = Delete From Array(array=w780, length=w775, index=w778) -> (array with subset deleted=w777:string[])  [unwired: 1 out]
        n470 = Delete From Array(array=w779, length=w775, index=w778) -> (array with subset deleted=w776:cluster{"Table":string[][]}[])  [unwired: 1 out]
        n471 = Bundle By Name(cluster=w773, "FW names"=w777, "Pos Names"=w776) -> (w774:T13)
      }
      event "Save Button": Value Change {
        # "\"Filter Wheel Settings Simulation\":{\n    \"Addr\":\"\",\n    \"Filters\":[\n      {\n        \"Names\":[\"Y\",\"J\",\"H\",\"Open\"],\n        \"Relative Position\":[1,2,3,4],\n        \"Wheel Name\":\"YJH\"\n      },\n      {\n        \"Names\":[\"Z\",\"Narrow\",\"Dark\",\"Open\"],\n        \"Relative Position\":[1,2,3,4],\n        \"Wheel Name\":\"NarrowBand\"\n      }"
        # "Need to copy data from array to filter wheel info cluster"
        n472 = event-data() -> ()  [unwired: 1 in, 6 out]
        n473 = Unbundle By Name(w784) -> ("state"=w782:refnum<user-event>, "Filter Wheel ref"=w792:refnum<class "Filter Wheel.lvclass">, "Filter Wheel Info"=w789:T7, "FW names"=w791:string[], "Pos Names"=w790:cluster{"Table":string[][]}[])
        n474 = for {
          tunnel: w791 -> [w801] mode=indexing
          tunnel: w790 -> [w800] mode=indexing
          tunnel: [w793] -> w787 mode=indexing
          n475 = Unbundle(w800) -> ("Table"=w797:string[][])
          n476 = Index Array(array=w797, index (col)=0 ("disabled index (col)")) -> (element=w798:string[])  [unwired: 1 in]
          n477 = Index Array(array=w797, index (col)=1 ("disabled index (col)")) -> (element=w795:string[])  [unwired: 1 in]
          n478 = Decimal String To Number(string=w795) -> (number=w794:i32[])  [unwired: 2 in, 1 out]
          n479 = Bundle By Name(cluster=T8 {"Names"=[], "Relative Position"=[], "Wheel Name"=""} ("Cluster"), "Wheel Name"=w801, "Relative Position"=w794, "Names"=w798) -> (w793:T8)
        }
        n480 = Generate User Event(user event=w782, event data cluster="Show Filter Wheels" ("event data")) -> ()  [unwired: 2 in, 2 out]
        n481 = Array Size(array=w787) -> (size(s)=w788:i32)
        n482 = Bundle By Name(cluster=w789, "Num Wheels"=w788, "Filters"=w787) -> (w786:T7)
        n483 = call-dynamic "Write Filter Wheel Info.vi"("Filter Wheel Info"=w786, "Filter Wheel in"=w792) -> ("Filter Wheel out"=w781:refnum<class "Filter Wheel.lvclass">)  [unwired: 8 in, 1 out]
        n484 = Bundle By Name(cluster=w784, "Filter Wheel Info"=w786, "Filter Wheel ref"=w781) -> (w785:T13)
      }
      event "Restore Defaults": Value Change {
        n485 = event-data() -> ()  [unwired: 1 in, 6 out]
        n486 = Unbundle By Name(w804) -> ("state"=w803:refnum<user-event>)
        n487 = Generate User Event(user event=w803, event data cluster="init Prime" ("event data")) -> ()  [unwired: 2 in, 2 out]
      }
      event "Close": Value Change {
        n488 = event-data() -> ()  [unwired: 1 in, 2 out]
        n489 = Unbundle By Name(w808) -> ("state"=w807:refnum<user-event>)
        n490 = Generate User Event(user event=w807, event data cluster="Shutdown" ("event data")) -> ()  [unwired: 2 in, 2 out]
      }
    }
  }
  "Wheel Name" <- "Filter Wheel name"
